vi "Test SwitchesMirrors.vi"() -> ()   [LabVIEW 2014]
uses:
  support/Instrument Status.ctl
  Spectrometer/Laser.ctl
  Spectrometer/Spectrometer Config.ctl
  Spectrometer/Laser Settings.ctl
  Spectrometer/Filter.ctl
  Spectrometer/Grating Detector Settings.ctl
  Spectrometer/Grating.ctl
  Spectrometer/Detector.ctl
  Spectrometer/Acquisition Settings.ctl
  SwitchesMirrors Config.ctl
  SwitchesMirrors Status.ctl
  SwitchesMirrors Refnum.ctl
  Camera/Camera Config.ctl
  Camera/Camera Settings.ctl
  Stress Control/StressControl Config.ctl
  Parameter Analyzer/Parameter Analyzer Config.ctl
  Parameter Analyzer/Parameter Analyzer Integration Parameters.ctl
  Parameter Analyzer/Parameter Analyzer SMU Sweeping.ctl
  Parameter Analyzer/Parameter Analyzer Sweep Spacing.ctl
  Parameter Analyzer/Parameter Analyzer SMU Range.ctl
  Parameter Analyzer/Parameter Analyzer SMU Sampling.ctl
  Parameter Analyzer/Parameter Analyzer Sampling Parameters.ctl
  Parameter Analyzer/Parameter Analyzer Stop Sampling Conditions.ctl
  Switching Matrix/Switching Matrix Config.ctl
  XYZ Stage/XYZ Config.ctl
  XYZ Stage/XYZ Connection Settings.ctl
  XYZ Stage/XYZ Stage Control.ctl
  XYZ Stage/XYZ Coordinate Control.ctl
  Autofocus/AutoFocus Config.ctl
  Autofocus/ZScan.ctl
  <vilib>/Analysis/Matrix/Datatypes/RealMatrix.ctl
  Measurements/Strain Measurement/Strain Measurement Config.ctl
  Measurements/Plot Data/PlotData Config.ctl
  Measurements/Plot Data/Measurement.ctl
  Measurements/Plot Data/WhichInstrument.ctl
  Parameter Analyzer/Electrical Data.ctl
  Spectrometer/Spectral Data.ctl
  Measurements/Instrument Sequence/Instrument Steps.ctl
  Measurements/Instrument Sequence/Action.ctl
  Measurements/Instrument Sequence/Instrument List.ctl
  support/User Event - Stop/User Event - Stop.lvlib
  support/Message Queue/Message Queue.lvlib
  <vilib>/Analysis/Matrix/NI_Matrix.lvlib
panel:
  out "Instrument Status":T1
  out "Status Log":string
  in  "Video":bool
  in  "Laser":bool
  in  "Switches & Mirrors VISA Session":refnum<visa-resource-name>="COM1"
  in  "Use LaserVideo Relays":bool=TRUE
  out "Last Operation":string
  in  "Exit":bool
  # "LICENSED MATERIALS – PROPERTY OF IBM\nCopyright IBM Corp. 2016,\nALL RIGHTS RESERVED"
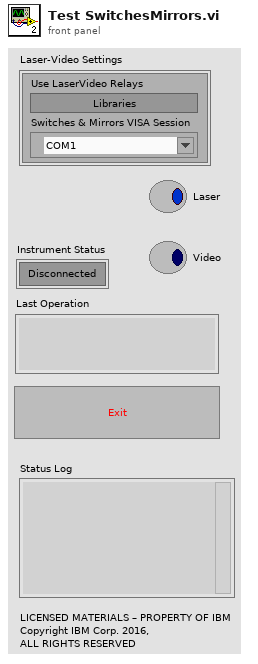
[diagram p1: front panel]
types:
  T1 = typedef "Instrument Status.ctl" = bool
  T2 = typedef "Message Queue.lvlib/All Message Queues.ctl" = cluster{"Message Handler Loop":refnum<queue>, "Parameter Analyzer":refnum<queue>, "Switching Matrix":refnum<queue>, "Stress Control":refnum<queue>, "Optical Spectrometer":refnum<queue>, "Switches & Mirrors":refnum<queue>, "Camera":refnum<queue>, "XYZ Stage":refnum<queue>, "AutoFocus":refnum<queue>, "Optoelectronic":refnum<queue>, "Save Data":refnum<queue>, "Plot Data":refnum<queue>, "Instrument Sequence":refnum<queue>, "Strain Measurement":refnum<queue>}
  T3 = typedef "Notifiers.ctl" = cluster{"Message Handler Loop":T4, "Parameter Analyzer":T5, "Switching Matrix":T6, "Stress Control":T7, "Optical Spectrometer":T8, "Switches & Mirrors":T9, "Camera":T10, "XYZ Stage":T11, "AutoFocus":T12, "Optoelectronic":T13, "Save Data":T14, "Plot Data":T14, "Instrument Sequence":T15, "Strain Measurement":cluster{"Status":refnum<notifier>, "Exit":refnum<notifier>, "Ready":refnum<notifier>}}
  T4 = typedef "Message Handler Loop Notifiers.ctl" = cluster{"Status":refnum<notifier>, "Instrument Data":refnum<notifier>, "Exit":refnum<notifier>, "Ready":refnum<notifier>}
  T5 = typedef "Parameter Analyzer Notifiers.ctl" = cluster{"Status":refnum<notifier>, "Instrument Data":refnum<notifier>, "Measurement":refnum<notifier>, "Exit":refnum<notifier>, "Ready":refnum<notifier>}
  T6 = typedef "Switching Matrix Notifiers.ctl" = cluster{"Status":refnum<notifier>, "Instrument Data":refnum<notifier>, "Measurement":refnum<notifier>, "Exit":refnum<notifier>, "Ready":refnum<notifier>}
  T7 = typedef "StressControl Notifiers.ctl" = cluster{"Status":refnum<notifier>, "Instrument Data":refnum<notifier>, "Measurement":refnum<notifier>, "Exit":refnum<notifier>, "Ready":refnum<notifier>}
  T8 = typedef "Spectrometer Notifiers.ctl" = cluster{"Status":refnum<notifier>, "Instrument Data":refnum<notifier>, "Measurement":refnum<notifier>, "Exit":refnum<notifier>, "Ready":refnum<notifier>}
  T9 = typedef "SwitchesMirrors Notifiers.ctl" = cluster{"Status":refnum<notifier>, "Instrument Data":refnum<notifier>, "Exit":refnum<notifier>, "Ready":refnum<notifier>}
  T10 = typedef "Camera Notifiers.ctl" = cluster{"Status":refnum<notifier>, "Instrument Data":refnum<notifier>, "Measurement":refnum<notifier>, "Exit":refnum<notifier>, "Ready":refnum<notifier>}
  T11 = typedef "XYZ Notifications.ctl" = cluster{"Status":refnum<notifier>, "Instrument Data":refnum<notifier>, "Measurement":refnum<notifier>, "Exit":refnum<notifier>, "Ready":refnum<notifier>}
  T12 = typedef "Autofocus Notifiers.ctl" = cluster{"Status":refnum<notifier>, "Instrument Data":refnum<notifier>, "Measurement":refnum<notifier>, "Exit":refnum<notifier>, "Ready":refnum<notifier>}
  T13 = typedef "Optoelectronic Notifiers.ctl" = cluster{"Status":refnum<notifier>, "Instrument Data":refnum<notifier>, "Measurement":refnum<notifier>, "Exit":refnum<notifier>, "Ready":refnum<notifier>}
  T14 = typedef "SaveData Notifiers.ctl" = cluster{"Status":refnum<notifier>, "Exit":refnum<notifier>, "Ready":refnum<notifier>}
  T15 = typedef "Instrument Sequence Notifiers.ctl" = cluster{"Status":refnum<notifier>, "Instrument Data":refnum<notifier>, "Measurement":refnum<notifier>, "Exit":refnum<notifier>, "Ready":refnum<notifier>}
  T16 = typedef "Configuration.ctl" = cluster{"Parameter Analizer":T17, "Switching Matrix":T25, "Stress Control":T26, "Optical Spectrometer":T27, "Switches & Mirrors":T35, "Camera":T37, "XYZ Stage":T39, "AutoFocus":T43, "Sava Data":T46, "PlotData":T51, "Instrument Sequence":T57, "Strain Measurement":T58}
  T17 = typedef "Parameter Analyzer Config.ctl" = cluster{"Parameter Analyzer VISA Session":refnum<visa-resource-name>, "Sweeping Time Parameters":T18, "Acquisition Mode":enum32{"Sweeping Mode", "Sampling Mode"}, "Status Polling Time (ms)":u32, "Comment":string, "SMU 1 - Sweeping":T19, "SMU 2 - Sweeping":T19, "SMU 3 - Sweeping":T19, "SMU 4 - Sweeping":T19, "Sweep Spacing":T20, "Range":T21, "SMU1 - Sampling":T22, "SMU2 - Sampling":T22, "SMU3 - Sampling":T22, "SMU4 - Sampling":T22, "Sampling Time Parameters":T23, "Stop Condition":T24}
  T18 = typedef "Parameter Analyzer Integration Parameters.ctl" = cluster{"Integration Time":u32, "Short Integration Time (s)":dbl, "Long Integration Time (s)":dbl, "Wait Time Parameter":dbl}
  T19 = typedef "Parameter Analyzer SMU Sweeping.ctl" = cluster{"Start / Offset":dbl, "Stop / Ratio":dbl, "Step \n(linear only)":dbl, "Compliance":dbl, "Power \nCompliance":dbl, "Mode":u32, "Function":i32, "Sweep Mode":bool}
  T20 = typedef "Parameter Analyzer Sweep Spacing.ctl" = u16
  T21 = typedef "Parameter Analyzer SMU Range.ctl" = u16
  T22 = typedef "Parameter Analyzer SMU Sampling.ctl" = cluster{"Source":dbl, "Compliance":dbl, "Mode":u32, "Function":bool}
  T23 = typedef "Parameter Analyzer Sampling Parameters.ctl" = cluster{"Initial Interval (s)":dbl, "Number of Samples":i32, "Total Sampling Time (s)":dbl, "Hold Time (s)":dbl, "Sampling Mode":i32, "Sampling Time":i32}
  T24 = typedef "Parameter Analyzer Stop Sampling Conditions.ctl" = cluster{"Enable Delay (s)":dbl, "Name":string, "Threshold":dbl, "num. of events":i32, "Event":i32, "Stop Condition Enable":bool}
  T25 = typedef "Switching Matrix Config.ctl" = cluster{"Switching Matrix VISA Session":refnum<visa-resource-name>, "Connections":cluster{"Connections":bool[], "Connection Type":enum16{"Disconnected", "Make - Break", "Break - Make"}}[]}
  T26 = typedef "StressControl Config.ctl" = cluster{"Stress Control VISA Session":refnum<visa-resource-name>, "Axis":i32, "Motion":u16, "Destination (°)":dbl, "Speed (°/s)":dbl, "Position (°)":dbl}
  T27 = typedef "Spectrometer Config.ctl" = cluster{"Laser Settings":T28, "Spectrometer Settings":T31, "Acquisition Settings":T34, "Path":path}
  T28 = typedef "Laser Settings.ctl" = cluster{"Laser Wavelength":T29, "Neutral Density Filter":T30}
  T29 = typedef "Laser.ctl" = enum16{"633 nm", "784 nm", "532 nm", "365 nm"}
  T30 = typedef "Filter.ctl" = enum16{"100%", "50%", "25%", "10%", "1%", "0.1%", "0.01%"}
  T31 = typedef "Grating Detector Settings.ctl" = cluster{"Confocal Hole Size (µm)":dbl, "Grating":T32, "Detector":T33}
  T32 = typedef "Grating.ctl" = u16
  T33 = typedef "Detector.ctl" = enum16{"InGaAs Array", "Silicon CCD"}
  T34 = typedef "Acquisition Settings.ctl" = cluster{"Acquisition Mode":enum16{"Single Window", "Multi-Window"}, "Spectal Position (nm)":dbl, "From (nm)":dbl, "To (nm)":dbl, "Integration Time (s)":dbl, "Number of Accumulations":i32, "AutoScanning":bool, "Spike Removal":bool}
  T35 = typedef "SwitchesMirrors Config.ctl" = cluster{"Relay VISA Session":refnum<visa-resource-name>, "Switches":T36, "Delays (ms)":cluster{"Laser":u32, "Video":u32}}
  T36 = typedef "SwitchesMirrors Status.ctl" = cluster{"Laser":bool, "Video":bool}
  T37 = typedef "Camera Config.ctl" = cluster{"Settings":T38}
  T38 = typedef "Camera Settings.ctl" = cluster{"Pixel clock":i32, "Frame rate":dbl, "Exposure time":dbl, "Master Gain":i32, "Red Gain":i32, "Green Gain":i32, "Blue Gain":i32, "Auto Gain":bool, "White-balance":bool, "Color Correction":bool}
  T39 = typedef "XYZ Config.ctl" = cluster{"Connection Settings":T40, "Manual Control":T41, "Coordinate Control":T42}
  T40 = typedef "XYZ Connection Settings.ctl" = cluster{"Tango VISA":refnum<visa-resource-name>, "Baudrate":i32, "Show Protocol?":bool}
  T41 = typedef "XYZ Stage Control.ctl" = cluster{"North":bool, "South":bool, "West":bool, "East":bool, "Up":bool, "Down":bool, "Stop":bool, "XY Step":dbl, "Z step":dbl}
  T42 = typedef "XYZ Coordinate Control.ctl" = cluster{"Motion Mode":enum16{"Absolute", "Relative"}, "Destination [mm]":dbl[]}
  T43 = typedef "AutoFocus Config.ctl" = cluster{"Matching Criteria":cluster{"Minimum Score":sgl, "Color Score Weight":sgl, "Minimum Contrast":i32, "Match Mode":u32, "Match Feature Mode":u32, "Subpixel Accuracy":bool, "Color Sensitivity":u32, "Search Strategy":u32}, "Z Scan Parameters":T44, "Displacement":dbl, "Transformation Matrix":T45}
  T44 = typedef "ZScan.ctl" = cluster{"Z Range":ext, "Resolution":dbl, "Initial Direction":enum16{"Up", "Down"}, "Focus Threshold":dbl, "Ascent Constant":dbl}
  T45 = typedef "NI_Matrix.lvlib/RealMatrix.ctl" = dbl[][]
  T46 = typedef "SaveData Config.ctl" = cluster{"Workspace Info":T47, "Instrument Configuration":T48, "Stress Motor Position":dbl, "Electrical Measurement":cluster{"Sequence":dbl[], "V1":dbl[], "V2":dbl[], "V3":dbl[], "V4":dbl[], "I1":dbl[], "I2":dbl[], "I3":dbl[], "I4":dbl[]}, "Optical Spectrum":T50}
  T47 = typedef "SaveData Workspace Info.ctl" = cluster{"Device Name":string, "Device Info":string, "Path":path}
  T48 = typedef "SaveData Instrument Configuration.ctl" = cluster{"Instrument":T49, "Configuration":string}
  T49 = typedef "Instrument List.ctl" = enum32{"Unknown Instrument", "Switching Matrix", "Parameter Analyzer", "Optical Spectrometer", "Optoelectronic", "Autofocus"}
  T50 = typedef "Spectral Data.ctl" = cluster{"Intensity":dbl[], "Wavelength":dbl[], "Energy":dbl[], "Raman Shift":dbl[], "Detector Temperature":dbl}
  T51 = typedef "PlotData Config.ctl" = cluster{"Sliders":cluster{"Strain Sequence":i32, "Instrument Sequence":i32}, "Measurement":T52, "Instrument Steps":T55, "Strain Points":dbl[]}
  T52 = typedef "Measurement.ctl" = cluster{"Which Instrument?":T53, "Electrical Measurement":T54, "Measurement Mode":enum16{"Sweeping Mode", "Sampling Mode"}, "Optical Spectrum":T50}
  T53 = typedef "WhichInstrument.ctl" = enum16{"No Plot", "Spectrometer", "Parameter Analyzer", "Optoelectronic"}
  T54 = typedef "Electrical Data.ctl" = cluster{"Sequence":dbl[], "V1":dbl[], "V2":dbl[], "V3":dbl[], "V4":dbl[], "I1":dbl[], "I2":dbl[], "I3":dbl[], "I4":dbl[]}
  T55 = typedef "Instrument Steps.ctl" = cluster{"Action":T56, "Configuration":variant, "Instrument":T49, "Status":enum8{"False", "True", "Mixed"}}[]
  T56 = typedef "Action.ctl" = enum32{"Configure", "Measure"}
  T57 = typedef "Instrument Sequence Config.ctl" = cluster{"Caller VI":enum16{"User", "Stress Measurement VI"}}
  T58 = typedef "Strain Measurement Config.ctl" = cluster{"Stress Sequence ":cluster{"Max Motor Position":ext, "# Intermediate Points":u32, "Initial Direction":enum16{"Tension", "Compression"}}, "Track?":bool}
  T59 = typedef "SwitchesMirrors Refnum.ctl" = cluster{"Instrument Status":refnum<vi>, "Laser":refnum<vi>, "Video":refnum<vi>, "Relay VISA":refnum<vi>}
  T60 = cluster{"SMU 1 - Sweeping":cluster{"Start / Offset":dbl, "Stop / Ratio":dbl, "Step (linear only)":dbl, "Compliance":dbl, "Power Compliance":dbl, "Mode":u32, "Function":i32, "Sweep Mode":bool}, "SMU 2 - Sweeping":cluster{"Start / Offset":dbl, "Stop / Ratio":dbl, "Step (linear only)":dbl, "Compliance":dbl, "Power Compliance":dbl, "Mode":u32, "Function":i32, "Sweep Mode":bool}, "SMU 3 - Sweeping":cluster{"Start / Offset":dbl, "Stop / Ratio":dbl, "Step (linear only)":dbl, "Compliance":dbl, "Power Compliance":dbl, "Mode":u32, "Function":i32, "Sweep Mode":bool}, "SMU 4 - Sweeping":cluster{"Start / Offset":dbl, "Stop / Ratio":dbl, "Step (linear only)":dbl, "Compliance":dbl, "Power Compliance":dbl, "Mode":u32, "Function":i32, "Sweep Mode":bool}, "Sweep Spacing":u16, "Range":u16}
  T61 = cluster{"SMU1 - Sampling":cluster{"Source":dbl, "Compliance":dbl, "Mode":u32, "Function":bool}, "SMU2 - Sampling":cluster{"Source":dbl, "Compliance":dbl, "Mode":u32, "Function":bool}, "SMU3 - Sampling":cluster{"Source":dbl, "Compliance":dbl, "Mode":u32, "Function":bool}, "SMU4 - Sampling":cluster{"Source":dbl, "Compliance":dbl, "Mode":u32, "Function":bool}, "Sampling Parameters":cluster{"Initial Interval (s)":dbl, "Number of Samples":i32, "Total Sampling Time (s)":dbl, "Hold Time (s)":dbl, "Sampling Mode":i32, "Sampling Time":i32}, "Stop Condition":cluster{"Enable Delay (s)":dbl, "Name":string, "Threshold":dbl, "num. of events":i32, "Event":i32, "Stop Condition Enable":bool}}
  T62 = cluster{"PlotData - Instrument Sequence":i32, "PlotData - Strain Sequence":i32}
  T63 = cluster{"Start / Offset":dbl, "Stop / Ratio":dbl, "Step (linear only)":dbl, "Compliance":dbl, "Power Compliance":dbl, "Mode":u32, "Function":i32, "Sweep Mode":bool}
  T64 = cluster{"Source":dbl, "Compliance":dbl, "Mode":u32, "Function":bool}
  T65 = cluster{"Initial Interval (s)":dbl, "Number of Samples":i32, "Total Sampling Time (s)":dbl, "Hold Time (s)":dbl, "Sampling Mode":i32, "Sampling Time":i32}
  T66 = cluster{"Enable Delay (s)":dbl, "Name":string, "Threshold":dbl, "num. of events":i32, "Event":i32, "Stop Condition Enable":bool}
  T67 = cluster{"Connections":bool[], "Connection Type":enum16{"Disconnected", "Make - Break", "Break - Make"}}[]
  T68 = cluster{"Minimum Score":sgl, "Color Score Weight":sgl, "Minimum Contrast":i32, "Match Mode":u32, "Match Feature Mode":u32, "Subpixel Accuracy":bool, "Color Sensitivity":u32, "Search Strategy":u32}
  T69 = cluster{"Max Motor Position":ext, "# Intermediate Points":u32, "Initial Direction":enum16{"Tension", "Compression"}}
  T70 = enum32{"invalid app kind", "Development System", "Run Time System", "Student Edition", "Embedded LabVIEW", "Evaluation", "Custom"}
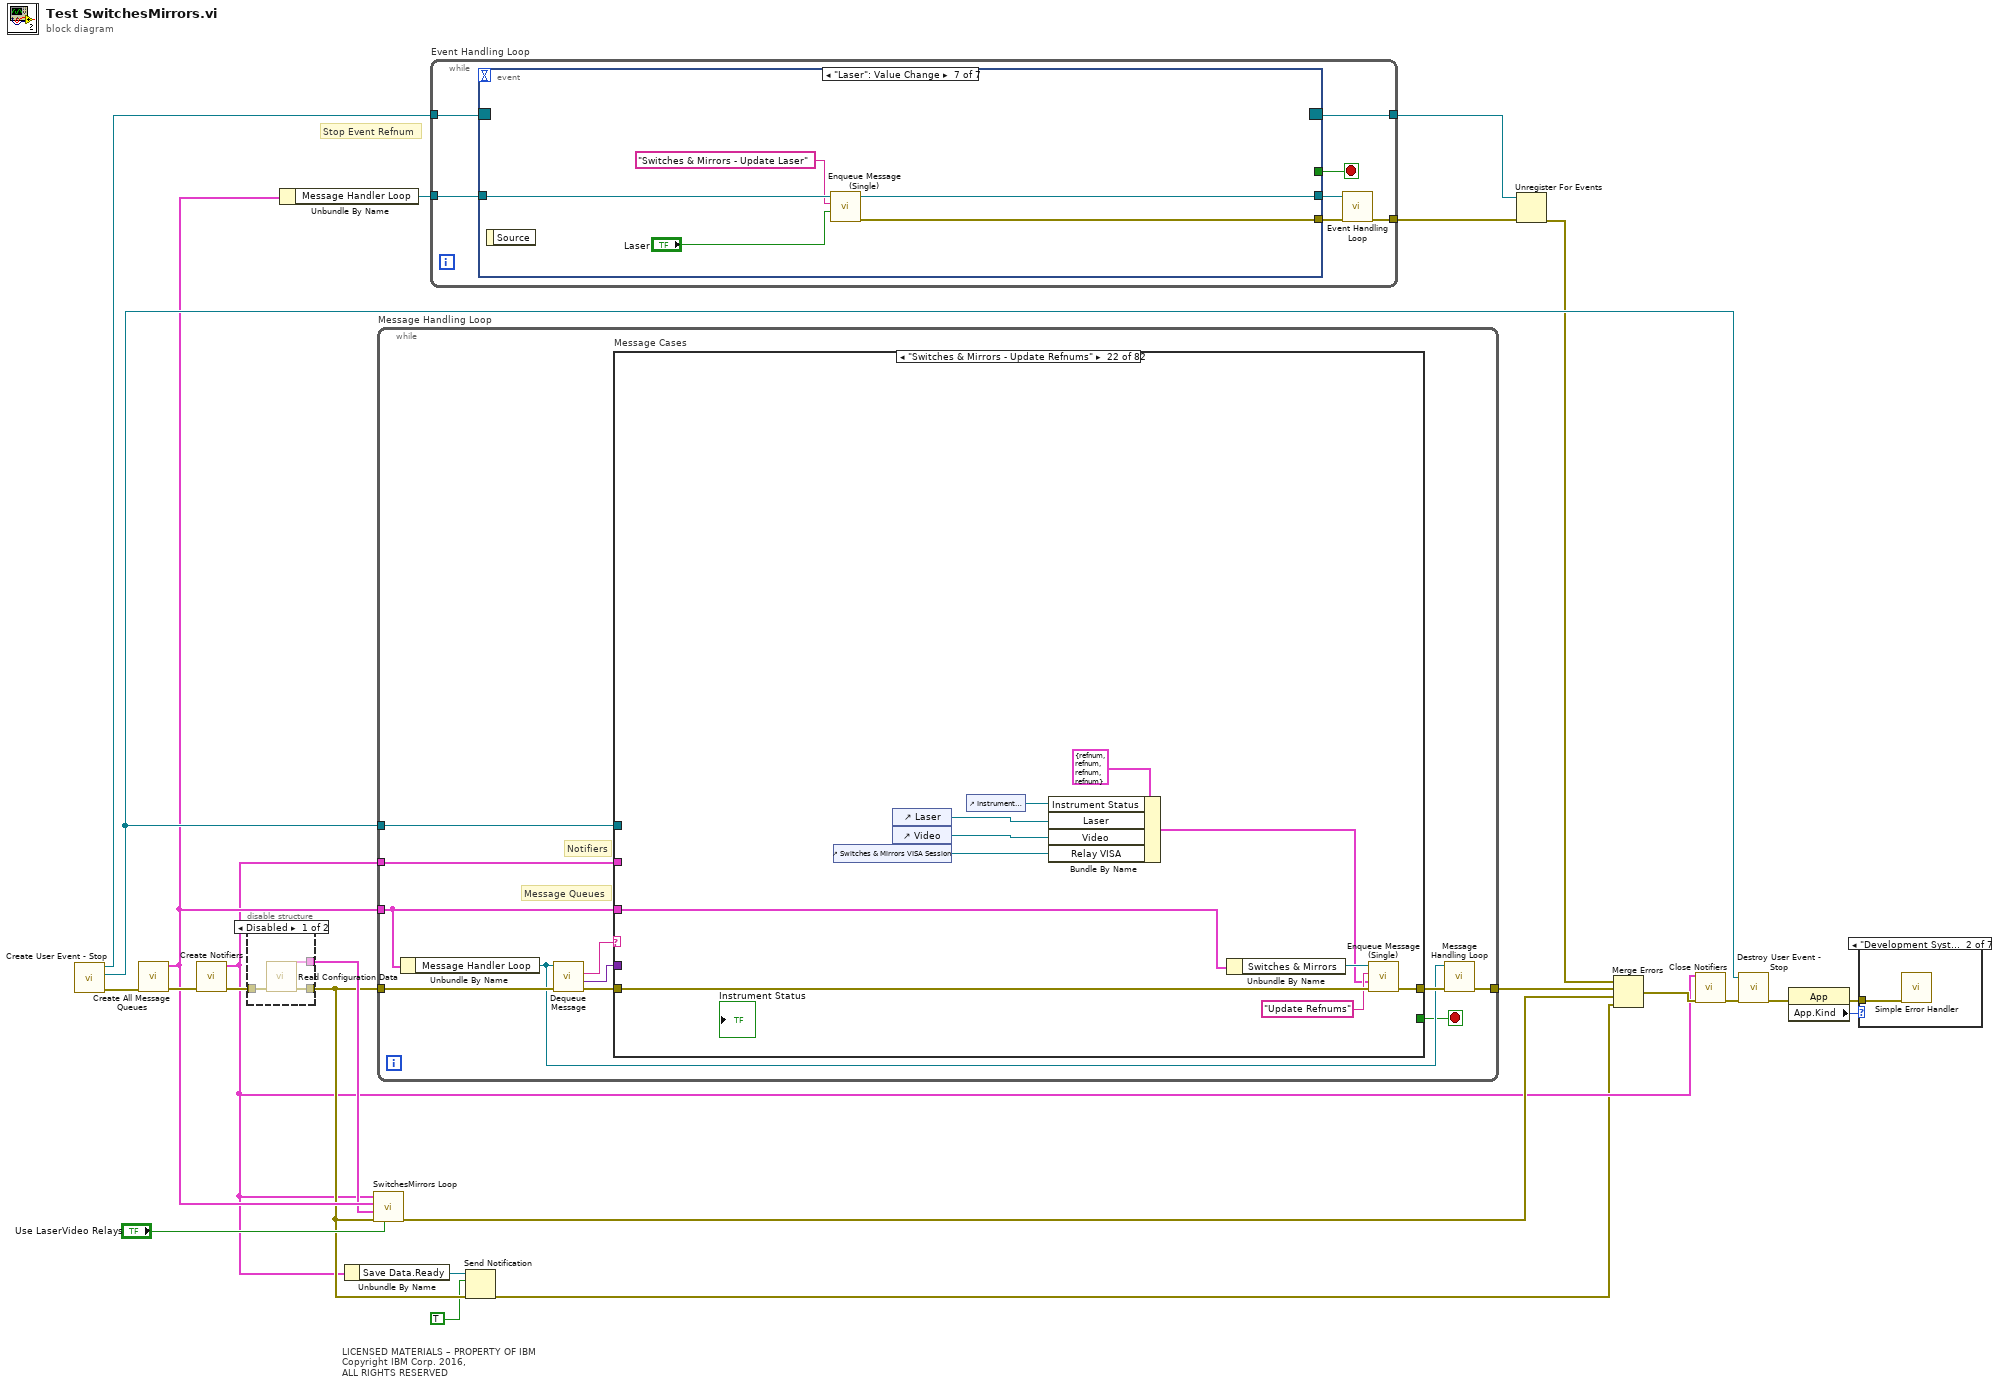
[diagram p0: block diagram]
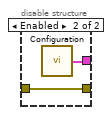
[diagram p2: hidden frame]
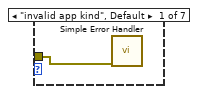
[diagram p3: hidden frame]
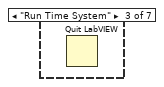
[diagram p4: hidden frame]
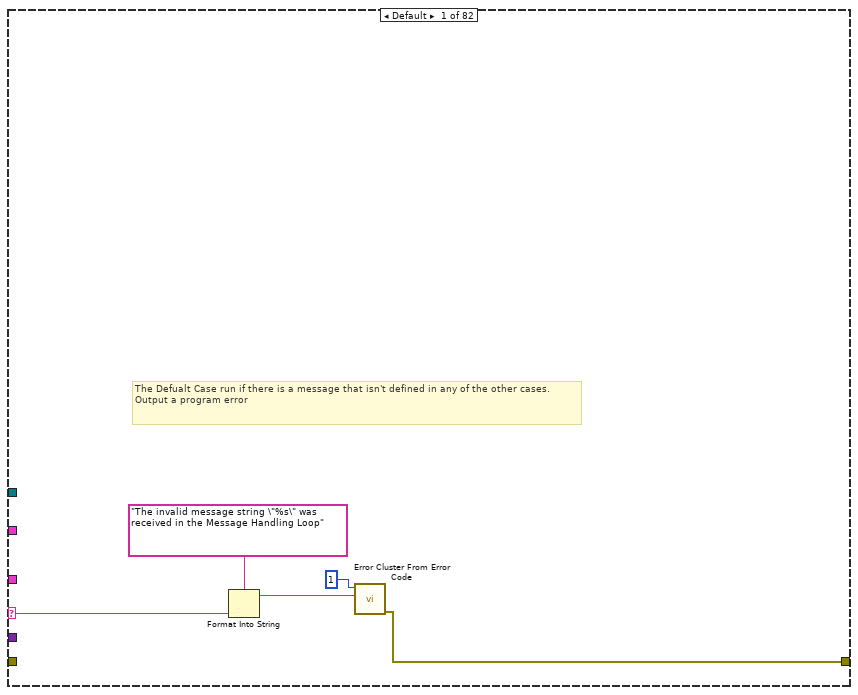
[diagram p9: hidden frame]
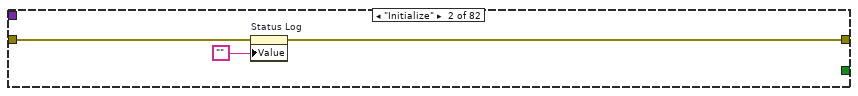
[diagram p10: hidden frame]
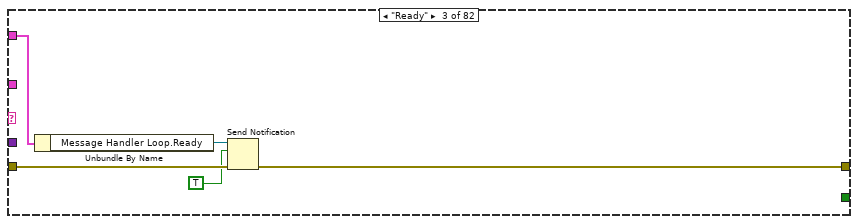
[diagram p11: hidden frame]
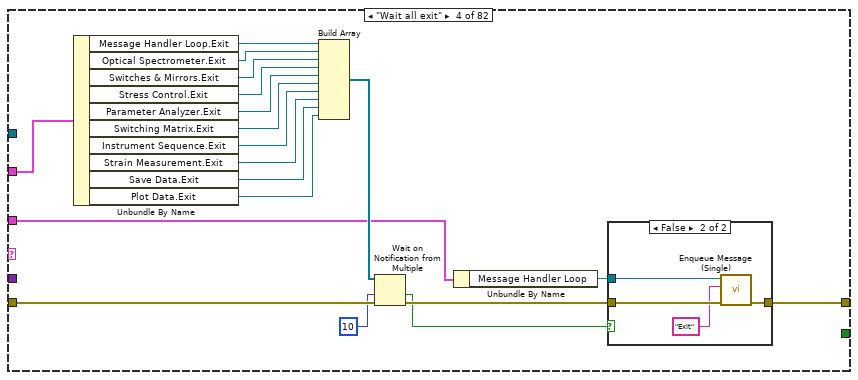
[diagram p12: hidden frame]
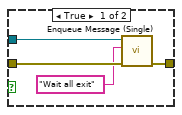
[diagram p13: hidden frame]
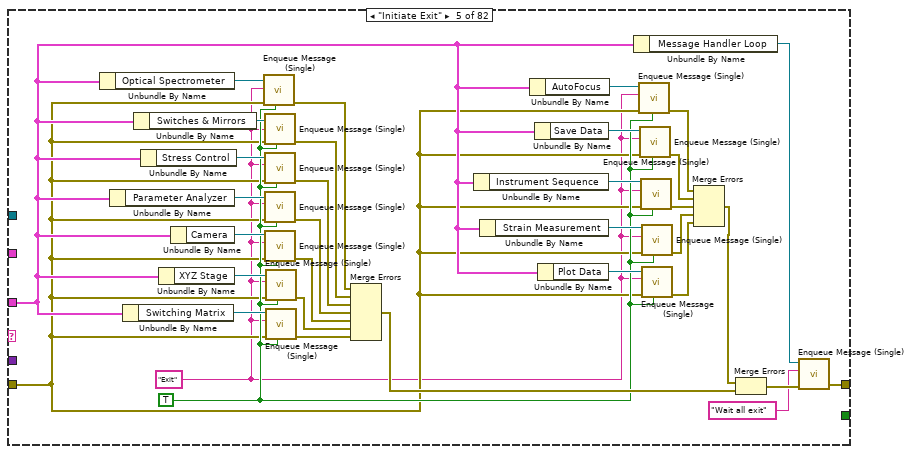
[diagram p14: hidden frame]
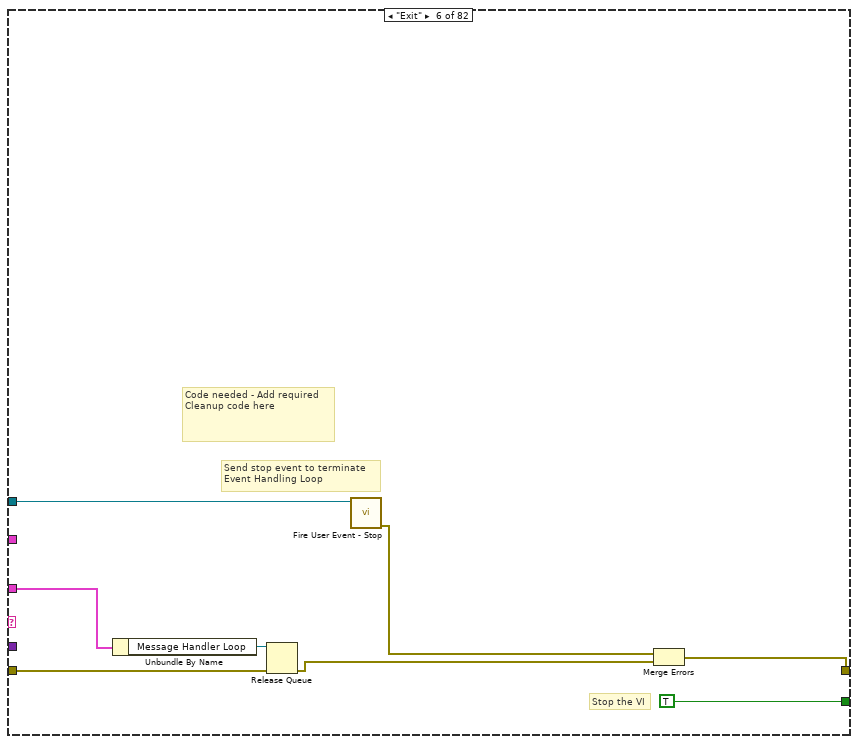
[diagram p15: hidden frame]
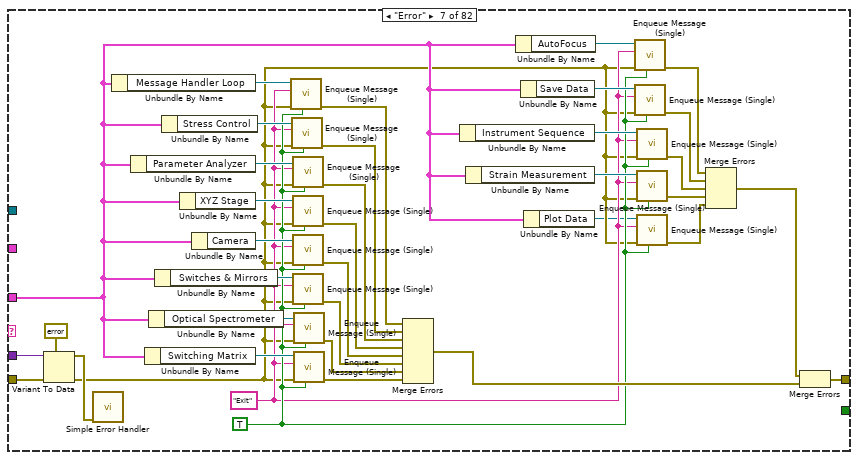
[diagram p16: hidden frame]
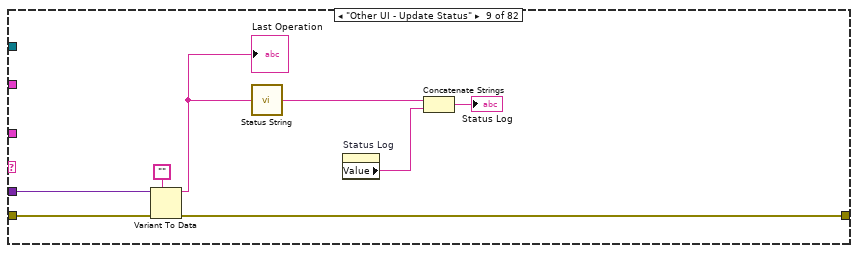
[diagram p18: hidden frame]
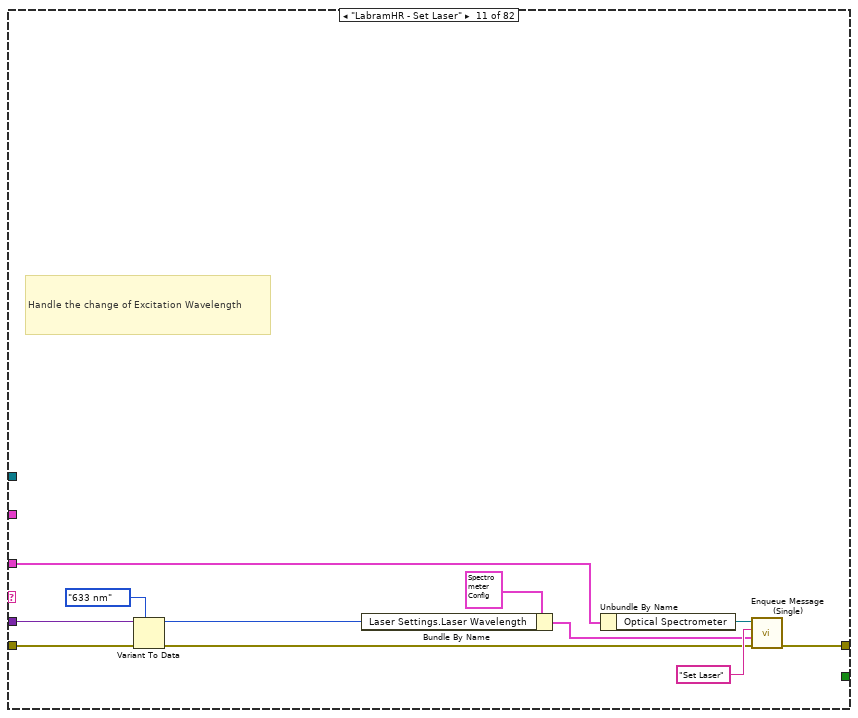
[diagram p20: hidden frame]
diagram:
  # "LICENSED MATERIALS – PROPERTY OF IBM\nCopyright IBM Corp. 2016,\nALL RIGHTS RESERVED"
  # "Stop Event Refnum"
  n1 = call "Create User Event - Stop.vi"() -> ("error out"=w14:errorcluster, "User Event - Stop"=w17:refnum<user-event>, "Stop Event Registration Refnum"=w24:refnum<event-registration>)  [unwired: 1 in, 8 out]
  n2 = call "Create All Message Queues.vi"("error in (no error)"=w14) -> ("error out"=w13:errorcluster, "Message Queues out"=w10:T2)  [unwired: 9 out]
  n3 = call "Create Notifiers.vi"("error in"=w13) -> ("error out"=w12:errorcluster, "Notifiers"=w4:T3)  [unwired: 9 out]
  n4 = disable-structure shown="Disabled" {
    disable-tunnel: w12 -> [w27 w29]
    disable-tunnel: [w26 w29] -> w5
    disable-tunnel: [w25 w28] -> w6
    frame Disabled {
      n5 = call "Read Configuration Data.vi"("error in"=w27) -> ("error out"=w26:errorcluster, "System Configuration"=w25:T16)  [unwired: 9 out]
    }
    frame Enabled {
      n6 = call "Configuration.vi"() -> ("IBM OptoElectroMechanics Configuration"=w28:T16)
    }
  }
  n7 = Unbundle By Name(w10) -> ("Message Handler Loop"=w22:refnum<queue>)
  n8 = Unbundle By Name(w4) -> ("Save Data.Ready"=w3:refnum<notifier>)
  n9 = call "SwitchesMirrors Loop.vi"("Used functions"="Use LaserVideo Relays", "error in"=w5, "IBM OptoElectroMechanics Configuration"=w6, "Message Queues out"=w10, "Notifiers"=w4) -> ("error out"=w7:errorcluster)  [unwired: 6 out]
  n10 = while "Message Handling Loop" {
    tunnel: w5 -> [w40]
    tunnel: [w37] -> w8
    tunnel: w10 -> [w31]
    tunnel: w17 -> [w33]
    tunnel: w4 -> [w30]
    stop <- w32 stop-if-true
    # "Notifiers"
    # "Message Queues"
    n11 = Unbundle By Name(w31) -> ("Message Handler Loop"=w36:refnum<queue>)
    n12 = call "Dequeue Message.vi"("error in (no error)"=w40, "Message Queue"=w36) -> ("error out"=w39:errorcluster, "Message Data"=w34:variant, "Message"=w35:string)  [unwired: 7 out]
    n13 = case "Message Cases" shown="\"Switches & Mirrors - Update Refnums\"" w35 {
      selector: w35 -> [w45 _ _ _ _ _ _ _ _ _ _ _ _ _ _ _ _ _ _ _ _ _ _ _ _ _ _ _ _ _ _ _ _ _ _ _ _ _ _ _ _ _ _ _ _ _ _ _ _ _ _ _ _ _ _ _ _ _ _ _ _ _ _ _ _ _ _ _ _ _ _ _ _ _ _ _ _ _ _ _ _ _]
      tunnel: w39 -> [_ w47 w52 w71 w84 w121 w148 w160 w168 w169 w176 w191 w202 w213 w224 w235 w246 w250 w255 w257 w265 w270 w284 w297 w308 w310 w320 w322 w327 w332 w343 w354 w355 w360 w364 w375 w386 w403 w420 w421 w426 w434 w445 w449 w454 w459 w470 w481 w482 w493 w504 w515 w516 w521 w526 w531 w536 w541 w546 w551 w556 w559 w564 w569 w574 w579 w582 w587 w592 w597 w608 w613 w618 w623 w626 w631 w636 w641 w646 w649 w662 w663]
      tunnel: [w41 w46 w53 w60 w100 w122 w157 w160 w165 w169 w174 w187 w198 w210 w221 w231 w244 w247 w252 w257 w261 w276 w287 w296 w307 w310 w319 w326 w331 w332 w342 w353 w359 w360 w363 w369 w381 w392 w412 w423 w426 w437 w448 w453 w458 w459 w465 w477 w482 w488 w499 w510 w519 w524 w529 w534 w539 w544 w549 w554 w556 w558 w563 w568 w573 w578 w584 w589 w594 w597 w605 w612 w617 w622 w625 w630 w635 w640 w645 w649 w657 w663] -> w38
      tunnel: w34 -> [_ _ _ _ _ _ w159 _ w167 _ w180 w190 w201 w212 w223 w234 w245 _ _ _ w260 _ w280 w298 w309 _ w321 _ _ _ w337 w348 _ _ w362 w374 w385 w402 w419 _ _ w431 w442 _ _ _ w469 w480 _ w492 w503 w514 _ _ _ _ _ _ _ _ _ _ _ _ _ _ _ _ _ _ w607 _ _ _ _ _ _ _ _ _ w661 _]
      tunnel: w33 -> [_ _ _ _ _ w119 _ _ _ _ _ _ _ _ _ _ _ _ _ _ _ _ _ _ _ _ _ _ _ _ _ _ _ _ _ _ _ _ _ _ _ _ _ _ _ _ _ _ _ _ _ _ _ _ _ _ _ _ _ _ _ _ _ _ _ _ _ _ _ _ _ _ _ _ _ _ _ _ _ _ _ _]
      tunnel: [_ _ _ _ _ TRUE _ _ _ _ _ _ _ _ _ _ _ _ _ _ _ _ _ _ _ _ _ _ _ _ _ _ _ _ _ _ _ _ _ _ _ _ _ _ _ _ _ _ _ _ _ _ _ _ _ _ _ _ _ _ _ _ _ _ _ _ _ _ _ _ _ _ _ _ _ _ _ _ _ _ _ _] -> w32
      tunnel: w31 -> [_ _ _ w59 w87 w116 w129 _ _ _ w179 w186 w195 w208 w219 w228 w240 w248 w253 _ _ w274 w285 w293 w304 _ w317 w324 w329 _ w339 w350 w357 _ _ w371 w380 w391 w411 w422 _ w435 w446 w451 w456 _ w464 w476 _ w487 w498 w509 w518 w523 w528 w533 w538 w543 w548 w553 _ w561 w566 w571 w576 w581 w586 w591 w596 _ w602 w609 w614 w619 w628 w633 w638 w643 w648 _ w656 _]
      tunnel: w30 -> [_ _ w51 w72 _ _ _ _ _ _ _ _ _ _ _ _ _ _ _ _ _ _ _ _ _ _ _ _ _ _ _ _ _ _ _ _ _ _ _ _ _ _ _ _ _ _ _ _ _ _ _ _ _ _ _ _ _ _ _ _ _ _ _ _ _ _ _ _ _ _ _ _ _ _ _ _ _ _ _ _ _ _]
      frame Default {
        # "The Defualt Case run if there is a message that isn't defined in any of the other cases.\nOutput a program error"
        n14 = Format Into String(format string="The invalid message string \"%s\" was  received in the Message Handling Loop", w45) -> (resulting string=w43:string)  [unwired: 2 in, 1 out]
        n15 = call <vilib>:"Error Cluster From Error Code.vi"("error message (\"\")"=w43, "error code (0)"=1) -> ("error out"=w41:errorcluster)  [unwired: 2 in, 5 out]
      }
      frame "Initialize" {
        n16 = property on="Status Log" class="Str"(error in=w47, "Value"="") -> (error out=w46:errorcluster)  [unwired: 1 in, 1 out]
      }
      frame "Ready" {
        n17 = Unbundle By Name(w51) -> ("Message Handler Loop.Ready"=w50:refnum<notifier>)
        n18 = Send Notification(notification=TRUE, notifier=w50, error in (no error)=w52) -> (error out=w53:errorcluster)  [unwired: 1 out]
      }
      frame "Wait all exit" {
        n19 = Unbundle By Name(w72) -> ("Message Handler Loop.Exit"=w69:refnum<notifier>, "Optical Spectrometer.Exit"=w68:refnum<notifier>, "Switches & Mirrors.Exit"=w67:refnum<notifier>, "Stress Control.Exit"=w66:refnum<notifier>, "Parameter Analyzer.Exit"=w65:refnum<notifier>, "Switching Matrix.Exit"=w64:refnum<notifier>, "Instrument Sequence.Exit"=w57:refnum<notifier>, "Strain Measurement.Exit"=w56:refnum<notifier>, "Save Data.Exit"=w55:refnum<notifier>, "Plot Data.Exit"=w54:refnum<notifier>)
        n20 = Build Array(w69, w68, w67, w66, w65, w64, w57, w56, w55, w54) -> (w63:refnum<notifier>[])
        n21 = Wait on Notification from Multiple(0:w63, 2:10 ("timeout in ms (-1)"), 3:w71) -> (10:w58:bool, 11:w61:errorcluster)  [unwired: 3 out]
        n22 = Unbundle By Name(w59) -> ("Message Handler Loop"=w62:refnum<queue>)
        n23 = case shown="False" w58 {
          tunnel: w62 -> [w76 w80]
          tunnel: w61 -> [w75 w79]
          tunnel: [w74 w78] -> w60
          frame True {
            n24 = call "Enqueue Message (Single).vi"("error in (no error)"=w75, "Message"="Wait all exit", "Message Queue"=w76) -> ("error out"=w74:errorcluster)  [unwired: 1 in, 7 out]
          }
          frame False {
            n25 = call "Enqueue Message (Single).vi"("error in (no error)"=w79, "Message"="Exit", "Message Queue"=w80) -> ("error out"=w78:errorcluster)  [unwired: 1 in, 7 out]
          }
        }
      }
      frame "Initiate Exit" {
        w85 = TRUE ("Priority Message? (F)")
        w82 = "Exit" ("Message")
        n26 = Unbundle By Name(w87) -> ("Optical Spectrometer"=w104:refnum<queue>)
        n27 = Unbundle By Name(w87) -> ("Parameter Analyzer"=w101:refnum<queue>)
        n28 = Unbundle By Name(w87) -> ("Switching Matrix"=w96:refnum<queue>)
        n29 = Unbundle By Name(w87) -> ("Switches & Mirrors"=w103:refnum<queue>)
        n30 = Unbundle By Name(w87) -> ("Stress Control"=w102:refnum<queue>)
        n31 = Unbundle By Name(w87) -> ("XYZ Stage"=w114:refnum<queue>)
        n32 = Unbundle By Name(w87) -> ("Camera"=w105:refnum<queue>)
        n33 = call "Enqueue Message (Single).vi"("Priority Message? (F)"=w85, "error in (no error)"=w84, "Message"=w82, "Message Queue"=w104) -> ("error out"=w106:errorcluster)  [unwired: 1 in, 6 out]
        n34 = call "Enqueue Message (Single).vi"("Priority Message? (F)"=w85, "error in (no error)"=w84, "Message"=w82, "Message Queue"=w103) -> ("error out"=w107:errorcluster)  [unwired: 1 in, 6 out]
        n35 = call "Enqueue Message (Single).vi"("Priority Message? (F)"=w85, "error in (no error)"=w84, "Message"=w82, "Message Queue"=w102) -> ("error out"=w108:errorcluster)  [unwired: 1 in, 6 out]
        n36 = call "Enqueue Message (Single).vi"("Priority Message? (F)"=w85, "error in (no error)"=w84, "Message"=w82, "Message Queue"=w101) -> ("error out"=w109:errorcluster)  [unwired: 1 in, 6 out]
        n37 = call "Enqueue Message (Single).vi"("Priority Message? (F)"=w85, "error in (no error)"=w84, "Message"=w82, "Message Queue"=w105) -> ("error out"=w110:errorcluster)  [unwired: 1 in, 6 out]
        n38 = call "Enqueue Message (Single).vi"("Priority Message? (F)"=w85, "error in (no error)"=w84, "Message"=w82, "Message Queue"=w114) -> ("error out"=w111:errorcluster)  [unwired: 1 in, 6 out]
        n39 = call "Enqueue Message (Single).vi"("Priority Message? (F)"=w85, "error in (no error)"=w84, "Message"=w82, "Message Queue"=w96) -> ("error out"=w112:errorcluster)  [unwired: 1 in, 6 out]
        n40 = Merge Errors(w106, w107, w108, w109, w110, w111, w112) -> (w113:errorcluster)
        n41 = Unbundle By Name(w87) -> ("Instrument Sequence"=w93:refnum<queue>)
        n42 = Unbundle By Name(w87) -> ("Strain Measurement"=w89:refnum<queue>)
        n43 = Unbundle By Name(w87) -> ("AutoFocus"=w95:refnum<queue>)
        n44 = Unbundle By Name(w87) -> ("Save Data"=w94:refnum<queue>)
        n45 = Unbundle By Name(w87) -> ("Plot Data"=w86:refnum<queue>)
        n46 = Unbundle By Name(w87) -> ("Message Handler Loop"=w98:refnum<queue>)
        n47 = call "Enqueue Message (Single).vi"("Priority Message? (F)"=w85, "error in (no error)"=w84, "Message"=w82, "Message Queue"=w95) -> ("error out"=w92:errorcluster)  [unwired: 1 in, 6 out]
        n48 = call "Enqueue Message (Single).vi"("Priority Message? (F)"=w85, "error in (no error)"=w84, "Message"=w82, "Message Queue"=w94) -> ("error out"=w91:errorcluster)  [unwired: 1 in, 6 out]
        n49 = call "Enqueue Message (Single).vi"("Priority Message? (F)"=w85, "error in (no error)"=w84, "Message"=w82, "Message Queue"=w93) -> ("error out"=w90:errorcluster)  [unwired: 1 in, 6 out]
        n50 = call "Enqueue Message (Single).vi"("Priority Message? (F)"=w85, "error in (no error)"=w84, "Message"=w82, "Message Queue"=w89) -> ("error out"=w88:errorcluster)  [unwired: 1 in, 6 out]
        n51 = call "Enqueue Message (Single).vi"("Priority Message? (F)"=w85, "error in (no error)"=w84, "Message"=w82, "Message Queue"=w86) -> ("error out"=w83:errorcluster)  [unwired: 1 in, 6 out]
        n52 = Merge Errors(w92, w91, w90, w88, w83) -> (w81:errorcluster)
        n53 = Merge Errors(w81, w113) -> (w99:errorcluster)
        n54 = call "Enqueue Message (Single).vi"("error in (no error)"=w99, "Message"="Wait all exit", "Message Queue"=w98) -> ("error out"=w100:errorcluster)  [unwired: 1 in, 7 out]
      }
      frame "Exit" {
        # "Send stop event to terminate \nEvent Handling Loop"
        # "Stop the VI"
        # "Code needed - Add required Cleanup code here"
        n55 = Unbundle By Name(w116) -> ("Message Handler Loop"=w115:refnum<queue>)
        n56 = Release Queue(queue=w115, error in (no error)=w121) -> (error out=w120:errorcluster)  [unwired: 3 out]
        n57 = call "Fire User Event - Stop.vi"("User Event - Stop"=w119) -> ("error out"=w118:errorcluster)  [unwired: 1 in, 9 out]
        n58 = Merge Errors(w118, w120) -> (w122:errorcluster)
      }
      frame "Error" {
        w128 = TRUE ("Priority Message? (F)")
        w127 = "Exit" ("Message")
        n59 = Variant To Data(error in=w148, type=errorcluster {"status"=FALSE, "code"=0, "source"=""} ("error out"), Variant=w159) -> (data=w156:errorcluster, error out=w125:errorcluster)
        n60 = call <vilib>:"Simple Error Handler.vi"("error in (no error)"=w156) -> ()  [unwired: 1 in, 8 out]
        n61 = Unbundle By Name(w129) -> ("Message Handler Loop"=w139:refnum<queue>)
        n62 = Unbundle By Name(w129) -> ("Parameter Analyzer"=w154:refnum<queue>)
        n63 = Unbundle By Name(w129) -> ("Switching Matrix"=w149:refnum<queue>)
        n64 = Unbundle By Name(w129) -> ("Optical Spectrometer"=w150:refnum<queue>)
        n65 = Unbundle By Name(w129) -> ("Switches & Mirrors"=w140:refnum<queue>)
        n66 = Unbundle By Name(w129) -> ("Stress Control"=w153:refnum<queue>)
        n67 = Unbundle By Name(w129) -> ("XYZ Stage"=w155:refnum<queue>)
        n68 = Unbundle By Name(w129) -> ("Camera"=w141:refnum<queue>)
        n69 = call "Enqueue Message (Single).vi"("Priority Message? (F)"=w128, "error in (no error)"=w125, "Message"=w127, "Message Queue"=w139) -> ("error out"=w138:errorcluster)  [unwired: 1 in, 6 out]
        n70 = call "Enqueue Message (Single).vi"("Priority Message? (F)"=w128, "error in (no error)"=w125, "Message"=w127, "Message Queue"=w153) -> ("error out"=w147:errorcluster)  [unwired: 1 in, 6 out]
        n71 = call "Enqueue Message (Single).vi"("Priority Message? (F)"=w128, "error in (no error)"=w125, "Message"=w127, "Message Queue"=w154) -> ("error out"=w146:errorcluster)  [unwired: 1 in, 6 out]
        n72 = call "Enqueue Message (Single).vi"("Priority Message? (F)"=w128, "error in (no error)"=w125, "Message"=w127, "Message Queue"=w155) -> ("error out"=w145:errorcluster)  [unwired: 1 in, 6 out]
        n73 = call "Enqueue Message (Single).vi"("Priority Message? (F)"=w128, "error in (no error)"=w125, "Message"=w127, "Message Queue"=w141) -> ("error out"=w144:errorcluster)  [unwired: 1 in, 6 out]
        n74 = call "Enqueue Message (Single).vi"("Priority Message? (F)"=w128, "error in (no error)"=w125, "Message"=w127, "Message Queue"=w140) -> ("error out"=w143:errorcluster)  [unwired: 1 in, 6 out]
        n75 = call "Enqueue Message (Single).vi"("Priority Message? (F)"=w128, "error in (no error)"=w125, "Message"=w127, "Message Queue"=w150) -> ("error out"=w152:errorcluster)  [unwired: 1 in, 6 out]
        n76 = call "Enqueue Message (Single).vi"("Priority Message? (F)"=w128, "error in (no error)"=w125, "Message"=w127, "Message Queue"=w149) -> ("error out"=w151:errorcluster)  [unwired: 1 in, 6 out]
        n77 = Merge Errors(w138, w147, w146, w145, w144, w143, w152, w151) -> (w142:errorcluster)
        n78 = Unbundle By Name(w129) -> ("Instrument Sequence"=w135:refnum<queue>)
        n79 = Unbundle By Name(w129) -> ("Strain Measurement"=w131:refnum<queue>)
        n80 = Unbundle By Name(w129) -> ("AutoFocus"=w137:refnum<queue>)
        n81 = Unbundle By Name(w129) -> ("Save Data"=w136:refnum<queue>)
        n82 = Unbundle By Name(w129) -> ("Plot Data"=w124:refnum<queue>)
        n83 = call "Enqueue Message (Single).vi"("Priority Message? (F)"=w128, "error in (no error)"=w125, "Message"=w127, "Message Queue"=w137) -> ("error out"=w132:errorcluster)  [unwired: 1 in, 6 out]
        n84 = call "Enqueue Message (Single).vi"("Priority Message? (F)"=w128, "error in (no error)"=w125, "Message"=w127, "Message Queue"=w136) -> ("error out"=w133:errorcluster)  [unwired: 1 in, 6 out]
        n85 = call "Enqueue Message (Single).vi"("Priority Message? (F)"=w128, "error in (no error)"=w125, "Message"=w127, "Message Queue"=w135) -> ("error out"=w134:errorcluster)  [unwired: 1 in, 6 out]
        n86 = call "Enqueue Message (Single).vi"("Priority Message? (F)"=w128, "error in (no error)"=w125, "Message"=w127, "Message Queue"=w131) -> ("error out"=w130:errorcluster)  [unwired: 1 in, 6 out]
        n87 = call "Enqueue Message (Single).vi"("Priority Message? (F)"=w128, "error in (no error)"=w125, "Message"=w127, "Message Queue"=w124) -> ("error out"=w126:errorcluster)  [unwired: 1 in, 6 out]
        n88 = Merge Errors(w132, w133, w134, w130, w126) -> (w123:errorcluster)
        n89 = Merge Errors(w123, w142) -> (w157:errorcluster)
      }
      frame "----- Other UI Events -----" {
        # "Other UI Events"
      }
      frame "Other UI - Update Status" {
        n90 = Variant To Data(error in=w168, type="", Variant=w167) -> (data=w161:string, error out=w165:errorcluster)
        "Last Operation" <- w161
        n91 = call "Status String.vi"("Message"=w161) -> ("Status String"=w164:string)
        n92 = property on="Status Log" class="Str"() -> ("Value"=w162:string)  [unwired: 2 in, 2 out]
        n93 = Concatenate Strings(w164, w162) -> (→"Status Log":string)
      }
      frame "----- Labram HR Events -----" {
        # "Labram HR Events"
      }
      frame "LabramHR - Set Laser" {
        # "Handle the change of Excitation Wavelength"
        n94 = Variant To Data(error in=w176, type=Laser."633 nm" ("NewVal"), Variant=w180) -> (data=w171:T29, error out=w175:errorcluster)
        n95 = Bundle By Name(cluster=T27 {"Laser Settings"={"Laser Wavelength"=enum."633 nm", "Neutral Density Filter"=enum."1%"}, "Spectrometer Settings"={"Confocal Hole Size (µm)"=150.0, "Grating"=1, "Detector"=enum."InGaAs Array"}, "Acquisition Settings"={"Acquisition Mode"=enum."Single Window", "Spectal Position (nm)"=480.0, "From (nm)"=632.0, "To (nm)"=1000.0, "Integration Time (s)"=3.0, "Number of Accumulations"=3, "AutoScanning"=FALSE, "Spike Removal"=FALSE}, "Path"=path ""} ("LabramHR"), "Laser Settings.Laser Wavelength"=w171) -> (w173:T27)
        n96 = Unbundle By Name(w179) -> ("Optical Spectrometer"=w178:refnum<queue>)
        n97 = call "Enqueue Message (Single).vi"("error in (no error)"=w175, "Message Data"=w173, "Message"="Set Laser", "Message Queue"=w178) -> ("error out"=w174:errorcluster)  [unwired: 7 out]
      }
      frame "LabramHR - Set Filter" {
        # "Handle the change of Neutral Density Filter"
        n98 = Variant To Data(error in=w191, type=Filter."1%" ("NewVal"), Variant=w190) -> (data=w182:T30, error out=w188:errorcluster)
        n99 = Bundle By Name(cluster=T27 {"Laser Settings"={"Laser Wavelength"=enum."633 nm", "Neutral Density Filter"=enum."1%"}, "Spectrometer Settings"={"Confocal Hole Size (µm)"=150.0, "Grating"=1, "Detector"=enum."InGaAs Array"}, "Acquisition Settings"={"Acquisition Mode"=enum."Single Window", "Spectal Position (nm)"=480.0, "From (nm)"=632.0, "To (nm)"=1000.0, "Integration Time (s)"=3.0, "Number of Accumulations"=3, "AutoScanning"=FALSE, "Spike Removal"=FALSE}, "Path"=path ""} ("LabramHR"), "Laser Settings.Neutral Density Filter"=w182) -> (w184:T27)
        n100 = Unbundle By Name(w186) -> ("Optical Spectrometer"=w189:refnum<queue>)
        n101 = call "Enqueue Message (Single).vi"("error in (no error)"=w188, "Message Data"=w184, "Message"="Set Filter", "Message Queue"=w189) -> ("error out"=w187:errorcluster)  [unwired: 7 out]
      }
      frame "LabramHR - Set Hole" {
        # "Handle the change in Confocal hole size"
        n102 = Variant To Data(error in=w202, type=150.0 ("Confocal Hole Size (µm) 2"), Variant=w201) -> (data=w194:dbl, error out=w197:errorcluster)
        n103 = Bundle By Name(cluster=T27 {"Laser Settings"={"Laser Wavelength"=enum."633 nm", "Neutral Density Filter"=enum."1%"}, "Spectrometer Settings"={"Confocal Hole Size (µm)"=150.0, "Grating"=1, "Detector"=enum."InGaAs Array"}, "Acquisition Settings"={"Acquisition Mode"=enum."Single Window", "Spectal Position (nm)"=480.0, "From (nm)"=632.0, "To (nm)"=1000.0, "Integration Time (s)"=3.0, "Number of Accumulations"=3, "AutoScanning"=FALSE, "Spike Removal"=FALSE}, "Path"=path ""} ("LabramHR"), "Spectrometer Settings.Confocal Hole Size (µm)"=w194) -> (w193:T27)
        n104 = Unbundle By Name(w195) -> ("Optical Spectrometer"=w199:refnum<queue>)
        n105 = call "Enqueue Message (Single).vi"("error in (no error)"=w197, "Message Data"=w193, "Message"="Set Hole", "Message Queue"=w199) -> ("error out"=w198:errorcluster)  [unwired: 7 out]
      }
      frame "LabramHR - Set Grating" {
        w204 = T32 1 items=["1800 l/mm", "150 l/mm"] ("NewVal")
        # "Handle the change of grating"
        n106 = Variant To Data(error in=w213, type=w204, Variant=w212) -> (data=w206:T32, error out=w209:errorcluster)
        n107 = Bundle By Name(cluster=T27 {"Laser Settings"={"Laser Wavelength"=enum."633 nm", "Neutral Density Filter"=enum."1%"}, "Spectrometer Settings"={"Confocal Hole Size (µm)"=150.0, "Grating"=1, "Detector"=enum."InGaAs Array"}, "Acquisition Settings"={"Acquisition Mode"=enum."Single Window", "Spectal Position (nm)"=480.0, "From (nm)"=632.0, "To (nm)"=1000.0, "Integration Time (s)"=3.0, "Number of Accumulations"=3, "AutoScanning"=FALSE, "Spike Removal"=FALSE}, "Path"=path ""} ("LabramHR"), "Spectrometer Settings.Grating"=w206) -> (w205:T27)
        n108 = Unbundle By Name(w208) -> ("Optical Spectrometer"=w211:refnum<queue>)
        n109 = call "Enqueue Message (Single).vi"("error in (no error)"=w209, "Message Data"=w205, "Message"="Set Grating", "Message Queue"=w211) -> ("error out"=w210:errorcluster)  [unwired: 7 out]
      }
      frame "LabramHR - Set Detector" {
        # "Handle the change of grating"
        n110 = Variant To Data(error in=w224, type=Detector."Silicon CCD" ("NewVal"), Variant=w223) -> (data=w217:T33, error out=w220:errorcluster)
        n111 = Bundle By Name(cluster=T27 {"Laser Settings"={"Laser Wavelength"=enum."633 nm", "Neutral Density Filter"=enum."1%"}, "Spectrometer Settings"={"Confocal Hole Size (µm)"=150.0, "Grating"=1, "Detector"=enum."InGaAs Array"}, "Acquisition Settings"={"Acquisition Mode"=enum."Single Window", "Spectal Position (nm)"=480.0, "From (nm)"=632.0, "To (nm)"=1000.0, "Integration Time (s)"=3.0, "Number of Accumulations"=3, "AutoScanning"=FALSE, "Spike Removal"=FALSE}, "Path"=path ""} ("LabramHR"), "Spectrometer Settings.Detector"=w217) -> (w216:T27)
        n112 = Unbundle By Name(w219) -> ("Optical Spectrometer"=w222:refnum<queue>)
        n113 = call "Enqueue Message (Single).vi"("error in (no error)"=w220, "Message Data"=w216, "Message"="Set Detector", "Message Queue"=w222) -> ("error out"=w221:errorcluster)  [unwired: 7 out]
      }
      frame "LabramHR - Set Spectal Position" {
        # "Handle the change of Spetrometer position"
        n114 = Variant To Data(error in=w235, type=480.0 ("Spectal Position (nm) 2"), Variant=w234) -> (data=w227:dbl, error out=w229:errorcluster)
        n115 = Bundle By Name(cluster=T27 {"Laser Settings"={"Laser Wavelength"=enum."633 nm", "Neutral Density Filter"=enum."1%"}, "Spectrometer Settings"={"Confocal Hole Size (µm)"=150.0, "Grating"=1, "Detector"=enum."InGaAs Array"}, "Acquisition Settings"={"Acquisition Mode"=enum."Single Window", "Spectal Position (nm)"=480.0, "From (nm)"=632.0, "To (nm)"=1000.0, "Integration Time (s)"=3.0, "Number of Accumulations"=3, "AutoScanning"=FALSE, "Spike Removal"=FALSE}, "Path"=path ""} ("LabramHR"), "Acquisition Settings.Spectal Position (nm)"=w227) -> (w226:T27)
        n116 = Unbundle By Name(w228) -> ("Optical Spectrometer"=w232:refnum<queue>)
        n117 = call "Enqueue Message (Single).vi"("error in (no error)"=w229, "Message Data"=w226, "Message"="Set Spectal Position", "Message Queue"=w232) -> ("error out"=w231:errorcluster)  [unwired: 7 out]
      }
      frame "LabramHR - Set Acquisition Settings" {
        # "Handle the change of integration time"
        n118 = Variant To Data(error in=w246, type=T34 {"Acquisition Mode"=enum."Single Window", "Spectal Position (nm)"=480.0, "From (nm)"=632.0, "To (nm)"=1000.0, "Integration Time (s)"=3.0, "Number of Accumulations"=3, "AutoScanning"=FALSE, "Spike Removal"=FALSE} ("Acquisition Settings 2"), Variant=w245) -> (data=w239:T34, error out=w243:errorcluster)
        n119 = Bundle By Name(cluster=T27 {"Laser Settings"={"Laser Wavelength"=enum."633 nm", "Neutral Density Filter"=enum."1%"}, "Spectrometer Settings"={"Confocal Hole Size (µm)"=150.0, "Grating"=1, "Detector"=enum."InGaAs Array"}, "Acquisition Settings"={"Acquisition Mode"=enum."Single Window", "Spectal Position (nm)"=480.0, "From (nm)"=632.0, "To (nm)"=1000.0, "Integration Time (s)"=3.0, "Number of Accumulations"=3, "AutoScanning"=FALSE, "Spike Removal"=FALSE}, "Path"=path ""} ("LabramHR"), "Acquisition Settings"=w239) -> (w238:T27)
        n120 = Unbundle By Name(w240) -> ("Optical Spectrometer"=w241:refnum<queue>)
        n121 = call "Enqueue Message (Single).vi"("error in (no error)"=w243, "Message Data"=w238, "Message"="Set Acquisition Settings", "Message Queue"=w241) -> ("error out"=w244:errorcluster)  [unwired: 7 out]
      }
      frame "LabramHR - Acquire Spectrum" {
        n122 = Unbundle By Name(w248) -> ("Optical Spectrometer"=w249:refnum<queue>)
        n123 = call "Enqueue Message (Single).vi"("error in (no error)"=w250, "Message"="Acquire Spectrum", "Message Queue"=w249) -> ("error out"=w247:errorcluster)  [unwired: 1 in, 7 out]
      }
      frame "LabramHR - Save Spectrum" {
        n124 = Unbundle By Name(w253) -> ("Optical Spectrometer"=w254:refnum<queue>)
        n125 = call "Enqueue Message (Single).vi"("error in (no error)"=w255, "Message"="Save Optical Spectrum", "Message Queue"=w254) -> ("error out"=w252:errorcluster)  [unwired: 1 in, 7 out]
      }
      frame "----- Switches & Mirrors Events -----" {
        # "Switches & Mirrors EVENTS"
      }
      frame "Switches & Mirrors - Set UI" {
        n126 = Variant To Data(error in=w265, type=T35 {"Relay VISA Session"="COM1", "Switches"={"Laser"=FALSE, "Video"=FALSE}, "Delays (ms)"={"Laser"=500, "Video"=1500}} ("Laser-Video Config"), Variant=w260) -> (data=w259:T35, error out=w261:errorcluster)
        n127 = Unbundle By Name(w259) -> ("Switches.Laser"=w264:bool, "Switches.Video"=w263:bool, "Relay VISA Session"=w262:refnum<visa-resource-name>)
        n128 = property on="Video" class="Bool (strict)"("Value"=w264) -> ()  [unwired: 2 in, 2 out]
        n129 = property on="Laser" class="Bool (strict)"("Value"=w263) -> ()  [unwired: 2 in, 2 out]
        n130 = property on="Switches & Mirrors VISA Session" class="VISAName"("Value"=w262) -> ()  [unwired: 2 in, 2 out]
      }
      frame "Switches & Mirrors - Update Refnums" {
        n131 = control-ref of="Switches & Mirrors VISA Session"() -> (w272:refnum<vi>)
        n132 = control-ref of="Laser"() -> (w273:refnum<vi>)
        n133 = control-ref of="Video"() -> (w271:refnum<vi>)
        n134 = control-ref of="Instrument Status"() -> (w266:refnum<vi>)
        n135 = Bundle By Name(cluster=T59 {"Instrument Status"=refnum, "Laser"=refnum, "Video"=refnum, "Relay VISA"=refnum} ("Laser Video Refnums"), "Instrument Status"=w266, "Laser"=w273, "Video"=w271, "Relay VISA"=w272) -> (w268:T59)
        n136 = Unbundle By Name(w274) -> ("Switches & Mirrors"=w275:refnum<queue>)
        n137 = call "Enqueue Message (Single).vi"("error in (no error)"=w270, "Message Data"=w268, "Message"="Update Refnums", "Message Queue"=w275) -> ("error out"=w276:errorcluster)  [unwired: 7 out]
      }
      frame "Switches & Mirrors - Update Visa Session" {
        n138 = Variant To Data(error in=w284, type=refnum<visa-resource-name> "COM1" ("Laser Video VISA Session 2"), Variant=w280) -> (data=w279:refnum<visa-resource-name>, error out=w282:errorcluster)
        n139 = Bundle By Name(cluster=T35 {"Relay VISA Session"="COM1", "Switches"={"Laser"=FALSE, "Video"=FALSE}, "Delays (ms)"={"Laser"=500, "Video"=1500}} ("Laser-Video Config"), "Relay VISA Session"=w279) -> (w278:T35)
        n140 = Unbundle By Name(w285) -> ("Switches & Mirrors"=w286:refnum<queue>)
        n141 = call "Enqueue Message (Single).vi"("error in (no error)"=w282, "Message Data"=w278, "Message"="Update VISA Session", "Message Queue"=w286) -> ("error out"=w287:errorcluster)  [unwired: 7 out]
      }
      frame "Switches & Mirrors - Update Laser" {
        n142 = Variant To Data(error in=w297, type=FALSE ("Laser"), Variant=w298) -> (data=w288:bool, error out=w295:errorcluster)
        n143 = Bundle By Name(cluster=T35 {"Relay VISA Session"="COM1", "Switches"={"Laser"=FALSE, "Video"=FALSE}, "Delays (ms)"={"Laser"=500, "Video"=1500}} ("Laser-Video Config"), "Switches.Laser"=w288) -> (w291:T35)
        n144 = Unbundle By Name(w293) -> ("Switches & Mirrors"=w294:refnum<queue>)
        n145 = call "Enqueue Message (Single).vi"("error in (no error)"=w295, "Message Data"=w291, "Message"="Update Laser", "Message Queue"=w294) -> ("error out"=w296:errorcluster)  [unwired: 7 out]
      }
      frame "Switches & Mirrors - Update Video" {
        n146 = Variant To Data(error in=w308, type=FALSE ("Laser"), Variant=w309) -> (data=w299:bool, error out=w306:errorcluster)
        n147 = Bundle By Name(cluster=T35 {"Relay VISA Session"="COM1", "Switches"={"Laser"=FALSE, "Video"=FALSE}, "Delays (ms)"={"Laser"=500, "Video"=1500}} ("Laser-Video Config"), "Switches.Video"=w299) -> (w302:T35)
        n148 = Unbundle By Name(w304) -> ("Switches & Mirrors"=w305:refnum<queue>)
        n149 = call "Enqueue Message (Single).vi"("error in (no error)"=w306, "Message Data"=w302, "Message"="Update Video", "Message Queue"=w305) -> ("error out"=w307:errorcluster)  [unwired: 7 out]
      }
      frame "----- Camera Events -----" {
        # "uEye Camera EVENTS"
      }
      frame "Camera - Update Settings" {
        w313 = T37 {"Settings"={"Pixel clock"=20, "Frame rate"=30.0, "Exposure time"=33.21525, "Master Gain"=0, "Red Gain"=0, "Green Gain"=0, "Blue Gain"=0, "Auto Gain"=FALSE, "White-balance"=FALSE, "Color Correction"=FALSE}} ("Camera Configuration")
        n150 = Unbundle By Name(w313) -> ("Settings"=w314:T38)
        n151 = Variant To Data(error in=w320, type=w314, Variant=w321) -> (data=w311:T38, error out=w315:errorcluster)
        n152 = Bundle By Name(cluster=w313, "Settings"=w311) -> (w312:T37)
        n153 = Unbundle By Name(w317) -> ("Camera"=w318:refnum<queue>)
        n154 = call "Enqueue Message (Single).vi"("error in (no error)"=w315, "Message Data"=w312, "Message"="Update Settings", "Message Queue"=w318) -> ("error out"=w319:errorcluster)  [unwired: 7 out]
      }
      frame "Camera - Start Live" {
        n155 = Unbundle By Name(w324) -> ("Camera"=w325:refnum<queue>)
        n156 = call "Enqueue Message (Single).vi"("error in (no error)"=w322, "Message"="Start Live", "Message Queue"=w325) -> ("error out"=w326:errorcluster)  [unwired: 1 in, 7 out]
      }
      frame "Camera - Stop Live" {
        n157 = Unbundle By Name(w329) -> ("Camera"=w330:refnum<queue>)
        n158 = call "Enqueue Message (Single).vi"("error in (no error)"=w327, "Message"="Stop Live", "Message Queue"=w330) -> ("error out"=w331:errorcluster)  [unwired: 1 in, 7 out]
      }
      frame "----- Stress Control Events -----" {
        # "Stress Control Events"
      }
      frame "Stress Control - Update Motion Mode" {
        w336 = u16 0 items=["Absolute", "Relative"] ("Motion 2")
        n159 = Variant To Data(error in=w343, type=w336, Variant=w337) -> (data=w335:u16, error out=w338:errorcluster)
        n160 = Bundle By Name(cluster=T26 {"Stress Control VISA Session"="", "Axis"=1, "Motion"=0, "Destination (°)"=0.0, "Speed (°/s)"=4.0, "Position (°)"=0.0} ("Stress Control Configuration"), "Motion"=w335) -> (w334:T26)
        n161 = Unbundle By Name(w339) -> ("Stress Control"=w340:refnum<queue>)
        n162 = call "Enqueue Message (Single).vi"("error in (no error)"=w338, "Message Data"=w334, "Message"="Update Motion Mode", "Message Queue"=w340) -> ("error out"=w342:errorcluster)  [unwired: 7 out]
      }
      frame "Stress Control - Update Destination" {
        n163 = Variant To Data(error in=w354, type=0.0 ("Destination (°) 2"), Variant=w348) -> (data=w347:dbl, error out=w349:errorcluster)
        n164 = Bundle By Name(cluster=T26 {"Stress Control VISA Session"="", "Axis"=1, "Motion"=0, "Destination (°)"=0.0, "Speed (°/s)"=4.0, "Position (°)"=0.0} ("Stress Control Configuration"), "Destination (°)"=w347) -> (w345:T26)
        n165 = Unbundle By Name(w350) -> ("Stress Control"=w351:refnum<queue>)
        n166 = call "Enqueue Message (Single).vi"("error in (no error)"=w349, "Message Data"=w345, "Message"="Update Destination", "Message Queue"=w351) -> ("error out"=w353:errorcluster)  [unwired: 7 out]
      }
      frame "Stress Control - Change Stress" {
        n167 = Unbundle By Name(w357) -> ("Stress Control"=w358:refnum<queue>)
        n168 = call "Enqueue Message (Single).vi"("error in (no error)"=w355, "Message"="Change Stress", "Message Queue"=w358) -> ("error out"=w359:errorcluster)  [unwired: 1 in, 7 out]
      }
      frame "----- Parameter Analyzer Events -----" {
        # "Parameter Analyzer Events"
      }
      frame "Parameter Analyzer - Set Settings" {
        n169 = Variant To Data(error in=w364, type=T17 {"Parameter Analyzer VISA Session"="COM1", "Sweeping Time Parameters"={"Integration Time"=0, "Short Integration Time (s)"=0.0, "Long Integration Time (s)"=0.0, "Wait Time Parameter"=1.0}, "Acquisition Mode"=enum."Sweeping Mode", "Status Polling Time (ms)"=1000, "Comment"="Test VI", "SMU 1 - Sweeping"={"Start / Offset"=0.0, "Stop / Ratio"=1.0, "Step \n(linear only)"=0.01, "Compliance"=0.1, "Power \nCompliance"=0.0, "Mode"=0, "Function"=0, "Sweep Mode"=FALSE}, "SMU 2 - Sweeping"={"Start / Offset"=0.0, "Stop / Ratio"=1.0, "Step \n(linear only)"=0.01, "Compliance"=0.1, "Power \nCompliance"=0.0, "Mode"=0, "Function"=0, "Sweep Mode"=FALSE}, "SMU 3 - Sweeping"={"Start / Offset"=0.0, "Stop / Ratio"=1.0, "Step \n(linear only)"=0.01, "Compliance"=0.1, "Power \nCompliance"=0.0, "Mode"=0, "Function"=0, "Sweep Mode"=FALSE}, "SMU 4 - Sweeping"={"Start / Offset"=0.0, "Stop / Ratio"=1.0, "Step \n(linear only)"=0.01, "Compliance"=0.1, "Power \nCompliance"=0.0, "Mode"=1, "Function"=0, "Sweep Mode"=FALSE}, "Sweep Spacing"=0, "Range"=0, "SMU1 - Sampling"={"Source"=10.0, "Compliance"=1e-05, "Mode"=0, "Function"=FALSE}, "SMU2 - Sampling"={"Source"=10.0, "Compliance"=1e-05, "Mode"=0, "Function"=FALSE}, "SMU3 - Sampling"={"Source"=10.0, "Compliance"=1e-05, "Mode"=0, "Function"=FALSE}, "SMU4 - Sampling"={"Source"=10.0, "Compliance"=1e-05, "Mode"=0, "Function"=FALSE}, "Sampling Time Parameters"={"Initial Interval (s)"=0.1, "Number of Samples"=60, "Total Sampling Time (s)"=10.0, "Hold Time (s)"=0.0, "Sampling Mode"=0, "Sampling Time"=0}, "Stop Condition"={"Enable Delay (s)"=0.0, "Name"="", "Threshold"=0.0, "num. of events"=1, "Event"=0, "Stop Condition Enable"=FALSE}} ("HP4155C Configuration"), Variant=w362) -> (error out=w363:errorcluster)  [unwired: 1 out]
      }
      frame "Parameter Analyzer - Update Visa Session" {
        w366 = T17 {"Parameter Analyzer VISA Session"="COM1", "Sweeping Time Parameters"={"Integration Time"=0, "Short Integration Time (s)"=0.0, "Long Integration Time (s)"=0.0, "Wait Time Parameter"=1.0}, "Acquisition Mode"=enum."Sweeping Mode", "Status Polling Time (ms)"=1000, "Comment"="Test VI", "SMU 1 - Sweeping"={"Start / Offset"=0.0, "Stop / Ratio"=1.0, "Step \n(linear only)"=0.01, "Compliance"=0.1, "Power \nCompliance"=0.0, "Mode"=0, "Function"=0, "Sweep Mode"=FALSE}, "SMU 2 - Sweeping"={"Start / Offset"=0.0, "Stop / Ratio"=1.0, "Step \n(linear only)"=0.01, "Compliance"=0.1, "Power \nCompliance"=0.0, "Mode"=0, "Function"=0, "Sweep Mode"=FALSE}, "SMU 3 - Sweeping"={"Start / Offset"=0.0, "Stop / Ratio"=1.0, "Step \n(linear only)"=0.01, "Compliance"=0.1, "Power \nCompliance"=0.0, "Mode"=0, "Function"=0, "Sweep Mode"=FALSE}, "SMU 4 - Sweeping"={"Start / Offset"=0.0, "Stop / Ratio"=1.0, "Step \n(linear only)"=0.01, "Compliance"=0.1, "Power \nCompliance"=0.0, "Mode"=1, "Function"=0, "Sweep Mode"=FALSE}, "Sweep Spacing"=0, "Range"=0, "SMU1 - Sampling"={"Source"=10.0, "Compliance"=1e-05, "Mode"=0, "Function"=FALSE}, "SMU2 - Sampling"={"Source"=10.0, "Compliance"=1e-05, "Mode"=0, "Function"=FALSE}, "SMU3 - Sampling"={"Source"=10.0, "Compliance"=1e-05, "Mode"=0, "Function"=FALSE}, "SMU4 - Sampling"={"Source"=10.0, "Compliance"=1e-05, "Mode"=0, "Function"=FALSE}, "Sampling Time Parameters"={"Initial Interval (s)"=0.1, "Number of Samples"=60, "Total Sampling Time (s)"=10.0, "Hold Time (s)"=0.0, "Sampling Mode"=0, "Sampling Time"=0}, "Stop Condition"={"Enable Delay (s)"=0.0, "Name"="", "Threshold"=0.0, "num. of events"=1, "Event"=0, "Stop Condition Enable"=FALSE}} ("HP4155C Configuration")
        n170 = Unbundle By Name(w366) -> ("Parameter Analyzer VISA Session"=w367:refnum<visa-resource-name>)
        n171 = Variant To Data(error in=w375, type=w367, Variant=w374) -> (data=w365:refnum<visa-resource-name>, error out=w370:errorcluster)
        n172 = Bundle By Name(cluster=w366, "Parameter Analyzer VISA Session"=w365) -> (w368:T17)
        n173 = Unbundle By Name(w371) -> ("Parameter Analyzer"=w372:refnum<queue>)
        n174 = call "Enqueue Message (Single).vi"("error in (no error)"=w370, "Message Data"=w368, "Message"="Update Visa Session", "Message Queue"=w372) -> ("error out"=w369:errorcluster)  [unwired: 7 out]
      }
      frame "Parameter Analyzer - Configure Integration time" {
        w376 = T17 {"Parameter Analyzer VISA Session"="COM1", "Sweeping Time Parameters"={"Integration Time"=0, "Short Integration Time (s)"=0.0, "Long Integration Time (s)"=0.0, "Wait Time Parameter"=1.0}, "Acquisition Mode"=enum."Sweeping Mode", "Status Polling Time (ms)"=1000, "Comment"="Test VI", "SMU 1 - Sweeping"={"Start / Offset"=0.0, "Stop / Ratio"=1.0, "Step \n(linear only)"=0.01, "Compliance"=0.1, "Power \nCompliance"=0.0, "Mode"=0, "Function"=0, "Sweep Mode"=FALSE}, "SMU 2 - Sweeping"={"Start / Offset"=0.0, "Stop / Ratio"=1.0, "Step \n(linear only)"=0.01, "Compliance"=0.1, "Power \nCompliance"=0.0, "Mode"=0, "Function"=0, "Sweep Mode"=FALSE}, "SMU 3 - Sweeping"={"Start / Offset"=0.0, "Stop / Ratio"=1.0, "Step \n(linear only)"=0.01, "Compliance"=0.1, "Power \nCompliance"=0.0, "Mode"=0, "Function"=0, "Sweep Mode"=FALSE}, "SMU 4 - Sweeping"={"Start / Offset"=0.0, "Stop / Ratio"=1.0, "Step \n(linear only)"=0.01, "Compliance"=0.1, "Power \nCompliance"=0.0, "Mode"=1, "Function"=0, "Sweep Mode"=FALSE}, "Sweep Spacing"=0, "Range"=0, "SMU1 - Sampling"={"Source"=10.0, "Compliance"=1e-05, "Mode"=0, "Function"=FALSE}, "SMU2 - Sampling"={"Source"=10.0, "Compliance"=1e-05, "Mode"=0, "Function"=FALSE}, "SMU3 - Sampling"={"Source"=10.0, "Compliance"=1e-05, "Mode"=0, "Function"=FALSE}, "SMU4 - Sampling"={"Source"=10.0, "Compliance"=1e-05, "Mode"=0, "Function"=FALSE}, "Sampling Time Parameters"={"Initial Interval (s)"=0.1, "Number of Samples"=60, "Total Sampling Time (s)"=10.0, "Hold Time (s)"=0.0, "Sampling Mode"=0, "Sampling Time"=0}, "Stop Condition"={"Enable Delay (s)"=0.0, "Name"="", "Threshold"=0.0, "num. of events"=1, "Event"=0, "Stop Condition Enable"=FALSE}} ("HP4155C Configuration")
        n175 = Unbundle By Name(w376) -> ("Sweeping Time Parameters"=w377:T18)
        n176 = Variant To Data(error in=w386, type=w377, Variant=w385) -> (data=w378:T18, error out=w382:errorcluster)
        n177 = Bundle By Name(cluster=w376, "Sweeping Time Parameters"=w378) -> (w379:T17)
        n178 = Unbundle By Name(w380) -> ("Parameter Analyzer"=w383:refnum<queue>)
        n179 = call "Enqueue Message (Single).vi"("error in (no error)"=w382, "Message Data"=w379, "Message"="Configure Integration Time", "Message Queue"=w383) -> ("error out"=w381:errorcluster)  [unwired: 7 out]
      }
      frame "Parameter Analyzer - Configure Sweeping" {
        n180 = Variant To Data(error in=w403, type=T60 {"SMU 1 - Sweeping"={"Start / Offset"=0.0, "Stop / Ratio"=0.0, "Step (linear only)"=0.0, "Compliance"=0.0, "Power Compliance"=0.0, "Mode"=0, "Function"=0, "Sweep Mode"=FALSE}, "SMU 2 - Sweeping"={"Start / Offset"=0.0, "Stop / Ratio"=0.0, "Step (linear only)"=0.0, "Compliance"=0.0, "Power Compliance"=0.0, "Mode"=0, "Function"=0, "Sweep Mode"=FALSE}, "SMU 3 - Sweeping"={"Start / Offset"=0.0, "Stop / Ratio"=0.0, "Step (linear only)"=0.0, "Compliance"=0.0, "Power Compliance"=0.0, "Mode"=0, "Function"=0, "Sweep Mode"=FALSE}, "SMU 4 - Sweeping"={"Start / Offset"=0.0, "Stop / Ratio"=0.0, "Step (linear only)"=0.0, "Compliance"=0.0, "Power Compliance"=0.0, "Mode"=0, "Function"=0, "Sweep Mode"=FALSE}, "Sweep Spacing"=0, "Range"=0} ("output cluster"), Variant=w402) -> (data=w401:T60, error out=w393:errorcluster)
        n181 = Unbundle By Name(w401) -> ("SMU 1 - Sweeping"=w396:T63, "SMU 2 - Sweeping"=w397:T63, "SMU 3 - Sweeping"=w398:T63, "SMU 4 - Sweeping"=w399:T63, "Sweep Spacing"=w400:u16, "Range"=w390:u16)
        n182 = Bundle By Name(cluster=T17 {"Parameter Analyzer VISA Session"="COM1", "Sweeping Time Parameters"={"Integration Time"=0, "Short Integration Time (s)"=0.0, "Long Integration Time (s)"=0.0, "Wait Time Parameter"=1.0}, "Acquisition Mode"=enum."Sweeping Mode", "Status Polling Time (ms)"=1000, "Comment"="Test VI", "SMU 1 - Sweeping"={"Start / Offset"=0.0, "Stop / Ratio"=1.0, "Step \n(linear only)"=0.01, "Compliance"=0.1, "Power \nCompliance"=0.0, "Mode"=0, "Function"=0, "Sweep Mode"=FALSE}, "SMU 2 - Sweeping"={"Start / Offset"=0.0, "Stop / Ratio"=1.0, "Step \n(linear only)"=0.01, "Compliance"=0.1, "Power \nCompliance"=0.0, "Mode"=0, "Function"=0, "Sweep Mode"=FALSE}, "SMU 3 - Sweeping"={"Start / Offset"=0.0, "Stop / Ratio"=1.0, "Step \n(linear only)"=0.01, "Compliance"=0.1, "Power \nCompliance"=0.0, "Mode"=0, "Function"=0, "Sweep Mode"=FALSE}, "SMU 4 - Sweeping"={"Start / Offset"=0.0, "Stop / Ratio"=1.0, "Step \n(linear only)"=0.01, "Compliance"=0.1, "Power \nCompliance"=0.0, "Mode"=1, "Function"=0, "Sweep Mode"=FALSE}, "Sweep Spacing"=0, "Range"=0, "SMU1 - Sampling"={"Source"=10.0, "Compliance"=1e-05, "Mode"=0, "Function"=FALSE}, "SMU2 - Sampling"={"Source"=10.0, "Compliance"=1e-05, "Mode"=0, "Function"=FALSE}, "SMU3 - Sampling"={"Source"=10.0, "Compliance"=1e-05, "Mode"=0, "Function"=FALSE}, "SMU4 - Sampling"={"Source"=10.0, "Compliance"=1e-05, "Mode"=0, "Function"=FALSE}, "Sampling Time Parameters"={"Initial Interval (s)"=0.1, "Number of Samples"=60, "Total Sampling Time (s)"=10.0, "Hold Time (s)"=0.0, "Sampling Mode"=0, "Sampling Time"=0}, "Stop Condition"={"Enable Delay (s)"=0.0, "Name"="", "Threshold"=0.0, "num. of events"=1, "Event"=0, "Stop Condition Enable"=FALSE}} ("HP4155C Configuration"), "SMU 1 - Sweeping"=w396, "SMU 2 - Sweeping"=w397, "SMU 3 - Sweeping"=w398, "SMU 4 - Sweeping"=w399, "Sweep Spacing"=w400, "Range"=w390) -> (w389:T17)
        n183 = Unbundle By Name(w391) -> ("Parameter Analyzer"=w394:refnum<queue>)
        n184 = call "Enqueue Message (Single).vi"("error in (no error)"=w393, "Message Data"=w389, "Message"="Configure Sweeping", "Message Queue"=w394) -> ("error out"=w392:errorcluster)  [unwired: 7 out]
      }
      frame "Parameter Analyzer - Configure Sampling" {
        n185 = Variant To Data(error in=w420, type=T61 {"SMU1 - Sampling"={"Source"=0.0, "Compliance"=0.0, "Mode"=0, "Function"=FALSE}, "SMU2 - Sampling"={"Source"=0.0, "Compliance"=0.0, "Mode"=0, "Function"=FALSE}, "SMU3 - Sampling"={"Source"=0.0, "Compliance"=0.0, "Mode"=0, "Function"=FALSE}, "SMU4 - Sampling"={"Source"=0.0, "Compliance"=0.0, "Mode"=0, "Function"=FALSE}, "Sampling Parameters"={"Initial Interval (s)"=0.0, "Number of Samples"=0, "Total Sampling Time (s)"=0.0, "Hold Time (s)"=0.0, "Sampling Mode"=0, "Sampling Time"=0}, "Stop Condition"={"Enable Delay (s)"=0.0, "Name"="", "Threshold"=0.0, "num. of events"=0, "Event"=0, "Stop Condition Enable"=FALSE}} ("output cluster"), Variant=w419) -> (data=w418:T61, error out=w413:errorcluster)
        n186 = Unbundle By Name(w418) -> ("SMU1 - Sampling"=w409:T64, "SMU2 - Sampling"=w408:T64, "SMU3 - Sampling"=w407:T64, "SMU4 - Sampling"=w406:T64, "Sampling Parameters"=w417:T65, "Stop Condition"=w416:T66)
        n187 = Bundle By Name(cluster=T17 {"Parameter Analyzer VISA Session"="COM1", "Sweeping Time Parameters"={"Integration Time"=0, "Short Integration Time (s)"=0.0, "Long Integration Time (s)"=0.0, "Wait Time Parameter"=1.0}, "Acquisition Mode"=enum."Sweeping Mode", "Status Polling Time (ms)"=1000, "Comment"="Test VI", "SMU 1 - Sweeping"={"Start / Offset"=0.0, "Stop / Ratio"=1.0, "Step \n(linear only)"=0.01, "Compliance"=0.1, "Power \nCompliance"=0.0, "Mode"=0, "Function"=0, "Sweep Mode"=FALSE}, "SMU 2 - Sweeping"={"Start / Offset"=0.0, "Stop / Ratio"=1.0, "Step \n(linear only)"=0.01, "Compliance"=0.1, "Power \nCompliance"=0.0, "Mode"=0, "Function"=0, "Sweep Mode"=FALSE}, "SMU 3 - Sweeping"={"Start / Offset"=0.0, "Stop / Ratio"=1.0, "Step \n(linear only)"=0.01, "Compliance"=0.1, "Power \nCompliance"=0.0, "Mode"=0, "Function"=0, "Sweep Mode"=FALSE}, "SMU 4 - Sweeping"={"Start / Offset"=0.0, "Stop / Ratio"=1.0, "Step \n(linear only)"=0.01, "Compliance"=0.1, "Power \nCompliance"=0.0, "Mode"=1, "Function"=0, "Sweep Mode"=FALSE}, "Sweep Spacing"=0, "Range"=0, "SMU1 - Sampling"={"Source"=10.0, "Compliance"=1e-05, "Mode"=0, "Function"=FALSE}, "SMU2 - Sampling"={"Source"=10.0, "Compliance"=1e-05, "Mode"=0, "Function"=FALSE}, "SMU3 - Sampling"={"Source"=10.0, "Compliance"=1e-05, "Mode"=0, "Function"=FALSE}, "SMU4 - Sampling"={"Source"=10.0, "Compliance"=1e-05, "Mode"=0, "Function"=FALSE}, "Sampling Time Parameters"={"Initial Interval (s)"=0.1, "Number of Samples"=60, "Total Sampling Time (s)"=10.0, "Hold Time (s)"=0.0, "Sampling Mode"=0, "Sampling Time"=0}, "Stop Condition"={"Enable Delay (s)"=0.0, "Name"="", "Threshold"=0.0, "num. of events"=1, "Event"=0, "Stop Condition Enable"=FALSE}} ("HP4155C Configuration"), "SMU1 - Sampling"=w409, "SMU2 - Sampling"=w408, "SMU3 - Sampling"=w407, "SMU4 - Sampling"=w406, "Sampling Time Parameters"=w417, "Stop Condition"=w416) -> (w410:T17)
        n188 = Unbundle By Name(w411) -> ("Parameter Analyzer"=w414:refnum<queue>)
        n189 = call "Enqueue Message (Single).vi"("error in (no error)"=w413, "Message Data"=w410, "Message"="Configure Sampling", "Message Queue"=w414) -> ("error out"=w412:errorcluster)  [unwired: 7 out]
      }
      frame "Parameter Analyzer - Save Measurement" {
        n190 = Unbundle By Name(w422) -> ("Parameter Analyzer"=w424:refnum<queue>)
        n191 = call "Enqueue Message (Single).vi"("error in (no error)"=w421, "Message"="Save Electrical Measurement", "Message Queue"=w424) -> ("error out"=w423:errorcluster)  [unwired: 1 in, 7 out]
      }
      frame "----- Switching Matrix Events ----- " {
        # "Switching Matrix Events"
      }
      frame "Switching Matrix - Update Visa Session" {
        w427 = T25 {"Switching Matrix VISA Session"="GPIB0::18::INSTR", "Connections"=[{"Connections"=[FALSE, FALSE, FALSE, FALSE, FALSE, FALSE, FALSE, FALSE, FALSE, FALSE, FALSE, FALSE], "Connection Type"=enum."Disconnected"}, {"Connections"=[FALSE, FALSE, FALSE, FALSE, FALSE, FALSE, FALSE, FALSE, FALSE, FALSE, FALSE, FALSE], "Connection Type"=enum."Disconnected"}, {"Connections"=[FALSE, FALSE, FALSE, FALSE, FALSE, FALSE, FALSE, FALSE, FALSE, FALSE, FALSE, FALSE], "Connection Type"=enum."Disconnected"}, {"Connections"=[FALSE, FALSE, FALSE, FALSE, FALSE, FALSE, FALSE, FALSE, FALSE, FALSE, FALSE, FALSE], "Connection Type"=enum."Disconnected"}, {"Connections"=[FALSE, FALSE, FALSE, FALSE, FALSE, FALSE, FALSE, FALSE, FALSE, FALSE, FALSE, FALSE], "Connection Type"=enum."Disconnected"}, {"Connections"=[FALSE, FALSE, FALSE, FALSE, FALSE, FALSE, FALSE, FALSE, FALSE, FALSE, FALSE, FALSE], "Connection Type"=enum."Disconnected"}, {"Connections"=[FALSE, FALSE, FALSE, FALSE, FALSE, FALSE, FALSE, FALSE, FALSE, FALSE, FALSE, FALSE], "Connection Type"=enum."Disconnected"}, {"Connections"=[FALSE, FALSE, FALSE, FALSE, FALSE, FALSE, FALSE, FALSE, FALSE, FALSE, FALSE, FALSE], "Connection Type"=enum."Disconnected"}]} ("Keythley 707A Switching Matrix Configuration")
        n192 = Unbundle By Name(w427) -> ("Switching Matrix VISA Session"=w428:refnum<visa-resource-name>)
        n193 = Variant To Data(error in=w434, type=w428, Variant=w431) -> (data=w430:refnum<visa-resource-name>, error out=w432:errorcluster)
        n194 = Bundle By Name(cluster=w427, "Switching Matrix VISA Session"=w430) -> (w429:T25)
        n195 = Unbundle By Name(w435) -> ("Switching Matrix"=w436:refnum<queue>)
        n196 = call "Enqueue Message (Single).vi"("error in (no error)"=w432, "Message Data"=w429, "Message"="Update Visa Session", "Message Queue"=w436) -> ("error out"=w437:errorcluster)  [unwired: 7 out]
      }
      frame "Switching Matrix - Set Connections" {
        w438 = T25 {"Switching Matrix VISA Session"="GPIB0::18::INSTR", "Connections"=[{"Connections"=[FALSE, FALSE, FALSE, FALSE, FALSE, FALSE, FALSE, FALSE, FALSE, FALSE, FALSE, FALSE], "Connection Type"=enum."Disconnected"}, {"Connections"=[FALSE, FALSE, FALSE, FALSE, FALSE, FALSE, FALSE, FALSE, FALSE, FALSE, FALSE, FALSE], "Connection Type"=enum."Disconnected"}, {"Connections"=[FALSE, FALSE, FALSE, FALSE, FALSE, FALSE, FALSE, FALSE, FALSE, FALSE, FALSE, FALSE], "Connection Type"=enum."Disconnected"}, {"Connections"=[FALSE, FALSE, FALSE, FALSE, FALSE, FALSE, FALSE, FALSE, FALSE, FALSE, FALSE, FALSE], "Connection Type"=enum."Disconnected"}, {"Connections"=[FALSE, FALSE, FALSE, FALSE, FALSE, FALSE, FALSE, FALSE, FALSE, FALSE, FALSE, FALSE], "Connection Type"=enum."Disconnected"}, {"Connections"=[FALSE, FALSE, FALSE, FALSE, FALSE, FALSE, FALSE, FALSE, FALSE, FALSE, FALSE, FALSE], "Connection Type"=enum."Disconnected"}, {"Connections"=[FALSE, FALSE, FALSE, FALSE, FALSE, FALSE, FALSE, FALSE, FALSE, FALSE, FALSE, FALSE], "Connection Type"=enum."Disconnected"}, {"Connections"=[FALSE, FALSE, FALSE, FALSE, FALSE, FALSE, FALSE, FALSE, FALSE, FALSE, FALSE, FALSE], "Connection Type"=enum."Disconnected"}]} ("Keythley 707A Switching Matrix Configuration")
        n197 = Unbundle By Name(w438) -> ("Connections"=w439:T67)
        n198 = Variant To Data(error in=w445, type=w439, Variant=w442) -> (data=w441:T67, error out=w443:errorcluster)
        n199 = Bundle By Name(cluster=w438, "Connections"=w441) -> (w440:T25)
        n200 = Unbundle By Name(w446) -> ("Switching Matrix"=w447:refnum<queue>)
        n201 = call "Enqueue Message (Single).vi"("error in (no error)"=w443, "Message Data"=w440, "Message"="Set Connections", "Message Queue"=w447) -> ("error out"=w448:errorcluster)  [unwired: 7 out]
      }
      frame "Switching Matrix - Disconnect All" {
        n202 = Unbundle By Name(w451) -> ("Switching Matrix"=w452:refnum<queue>)
        n203 = call "Enqueue Message (Single).vi"("error in (no error)"=w449, "Message"="Disconnect All", "Message Queue"=w452) -> ("error out"=w453:errorcluster)  [unwired: 1 in, 7 out]
      }
      frame "Switching Matrix - Ground All" {
        n204 = Unbundle By Name(w456) -> ("Switching Matrix"=w457:refnum<queue>)
        n205 = call "Enqueue Message (Single).vi"("error in (no error)"=w454, "Message"="Ground All", "Message Queue"=w457) -> ("error out"=w458:errorcluster)  [unwired: 1 in, 7 out]
      }
      frame "----- XYZ Stage Events -----" {
        # "NEW DEVICE EVENTS"
      }
      frame "XYZ Stage - Update Visa Session" {
        w460 = T39 {"Connection Settings"={"Tango VISA"="", "Baudrate"=57600, "Show Protocol?"=FALSE}, "Manual Control"={"North"=FALSE, "South"=FALSE, "West"=FALSE, "East"=FALSE, "Up"=FALSE, "Down"=FALSE, "Stop"=FALSE, "XY Step"=0.0, "Z step"=0.0}, "Coordinate Control"={"Motion Mode"=enum."Absolute", "Destination [mm]"=[]}} ("Configuration")
        n206 = Unbundle By Name(w460) -> ("Connection Settings.Tango VISA"=w468:refnum<visa-resource-name>)
        n207 = Variant To Data(error in=w470, type=w468, Variant=w469) -> (data=w461:refnum<visa-resource-name>, error out=w466:errorcluster)
        n208 = Bundle By Name(cluster=w460, "Connection Settings.Tango VISA"=w461) -> (w462:T39)
        n209 = Unbundle By Name(w464) -> ("XYZ Stage"=w463:refnum<queue>)
        n210 = call "Enqueue Message (Single).vi"("error in (no error)"=w466, "Message Data"=w462, "Message"="Manual Control", "Message Queue"=w463) -> ("error out"=w465:errorcluster)  [unwired: 7 out]
      }
      frame "XYZ Stage - Manual Control" {
        w472 = T39 {"Connection Settings"={"Tango VISA"="", "Baudrate"=57600, "Show Protocol?"=FALSE}, "Manual Control"={"North"=FALSE, "South"=FALSE, "West"=FALSE, "East"=FALSE, "Up"=FALSE, "Down"=FALSE, "Stop"=FALSE, "XY Step"=0.0, "Z step"=0.0}, "Coordinate Control"={"Motion Mode"=enum."Absolute", "Destination [mm]"=[]}} ("Configuration")
        n211 = Unbundle By Name(w472) -> ("Manual Control"=w471:T41)
        n212 = Variant To Data(error in=w481, type=w471, Variant=w480) -> (data=w473:T41, error out=w478:errorcluster)
        n213 = Bundle By Name(cluster=w472, "Manual Control"=w473) -> (w474:T39)
        n214 = Unbundle By Name(w476) -> ("XYZ Stage"=w475:refnum<queue>)
        n215 = call "Enqueue Message (Single).vi"("error in (no error)"=w478, "Message Data"=w474, "Message"="Manual Control", "Message Queue"=w475) -> ("error out"=w477:errorcluster)  [unwired: 7 out]
      }
      frame "----- AutoFocus Events -----" {
        # "NEW DEVICE EVENTS"
      }
      frame "AutoFocus - Set Match Criteria" {
        w483 = T43 {"Matching Criteria"={"Minimum Score"=700.0, "Color Score Weight"=57600.0, "Minimum Contrast"=50, "Match Mode"=0, "Match Feature Mode"=0, "Subpixel Accuracy"=TRUE, "Color Sensitivity"=1, "Search Strategy"=1}, "Z Scan Parameters"={"Z Range"=1380.0, "Resolution"=5000.0, "Initial Direction"=enum."Up", "Focus Threshold"=700.0, "Ascent Constant"=0.1}, "Displacement"=0.0, "Transformation Matrix"=[]} ("Configuration")
        n216 = Unbundle By Name(w483) -> ("Matching Criteria"=w491:T68)
        n217 = Variant To Data(error in=w493, type=w491, Variant=w492) -> (data=w484:T68, error out=w489:errorcluster)
        n218 = Bundle By Name(cluster=w483, "Matching Criteria"=w484) -> (w485:T43)
        n219 = Unbundle By Name(w487) -> ("AutoFocus"=w486:refnum<queue>)
        n220 = call "Enqueue Message (Single).vi"("error in (no error)"=w489, "Message Data"=w485, "Message"="Set Match Criteria", "Message Queue"=w486) -> ("error out"=w488:errorcluster)  [unwired: 7 out]
      }
      frame "AutoFocus - Link Stage & Camera" {
        w494 = T43 {"Matching Criteria"={"Minimum Score"=700.0, "Color Score Weight"=57600.0, "Minimum Contrast"=50, "Match Mode"=0, "Match Feature Mode"=0, "Subpixel Accuracy"=TRUE, "Color Sensitivity"=1, "Search Strategy"=1}, "Z Scan Parameters"={"Z Range"=1380.0, "Resolution"=5000.0, "Initial Direction"=enum."Up", "Focus Threshold"=700.0, "Ascent Constant"=0.1}, "Displacement"=0.0, "Transformation Matrix"=[]} ("Configuration")
        n221 = Unbundle By Name(w494) -> ("Displacement"=w502:dbl)
        n222 = Variant To Data(error in=w504, type=w502, Variant=w503) -> (data=w495:dbl, error out=w500:errorcluster)
        n223 = Bundle By Name(cluster=w494, "Displacement"=w495) -> (w496:T43)
        n224 = Unbundle By Name(w498) -> ("AutoFocus"=w497:refnum<queue>)
        n225 = call "Enqueue Message (Single).vi"("error in (no error)"=w500, "Message Data"=w496, "Message"="Link Stage & Camera", "Message Queue"=w497) -> ("error out"=w499:errorcluster)  [unwired: 7 out]
      }
      frame "AutoFocus - Focus" {
        w505 = T43 {"Matching Criteria"={"Minimum Score"=700.0, "Color Score Weight"=57600.0, "Minimum Contrast"=50, "Match Mode"=0, "Match Feature Mode"=0, "Subpixel Accuracy"=TRUE, "Color Sensitivity"=1, "Search Strategy"=1}, "Z Scan Parameters"={"Z Range"=1380.0, "Resolution"=5000.0, "Initial Direction"=enum."Up", "Focus Threshold"=700.0, "Ascent Constant"=0.1}, "Displacement"=0.0, "Transformation Matrix"=[]} ("Configuration")
        n226 = Unbundle By Name(w505) -> ("Z Scan Parameters"=w513:T44)
        n227 = Variant To Data(error in=w515, type=w513, Variant=w514) -> (data=w506:T44, error out=w511:errorcluster)
        n228 = Bundle By Name(cluster=w505, "Z Scan Parameters"=w506) -> (w507:T43)
        n229 = Unbundle By Name(w509) -> ("AutoFocus"=w508:refnum<queue>)
        n230 = call "Enqueue Message (Single).vi"("error in (no error)"=w511, "Message Data"=w507, "Message"="Focus", "Message Queue"=w508) -> ("error out"=w510:errorcluster)  [unwired: 7 out]
      }
      frame "AutoFocus - Set Target" {
        n231 = Unbundle By Name(w518) -> ("AutoFocus"=w517:refnum<queue>)
        n232 = call "Enqueue Message (Single).vi"("error in (no error)"=w516, "Message"="Set Target", "Message Queue"=w517) -> ("error out"=w519:errorcluster)  [unwired: 1 in, 7 out]
      }
      frame "AutoFocus - Find Target" {
        n233 = Unbundle By Name(w523) -> ("AutoFocus"=w522:refnum<queue>)
        n234 = call "Enqueue Message (Single).vi"("error in (no error)"=w521, "Message"="Find Target", "Message Queue"=w522) -> ("error out"=w524:errorcluster)  [unwired: 1 in, 7 out]
      }
      frame "AutoFocus - Align" {
        n235 = Unbundle By Name(w528) -> ("AutoFocus"=w527:refnum<queue>)
        n236 = call "Enqueue Message (Single).vi"("error in (no error)"=w526, "Message"="Align", "Message Queue"=w527) -> ("error out"=w529:errorcluster)  [unwired: 1 in, 7 out]
      }
      frame "AutoFocus - Grab Image" {
        n237 = Unbundle By Name(w533) -> ("AutoFocus"=w532:refnum<queue>)
        n238 = call "Enqueue Message (Single).vi"("error in (no error)"=w531, "Message"="Grab Image", "Message Queue"=w532) -> ("error out"=w534:errorcluster)  [unwired: 1 in, 7 out]
      }
      frame "AutoFocus - Set ROI" {
        n239 = Unbundle By Name(w538) -> ("AutoFocus"=w537:refnum<queue>)
        n240 = call "Enqueue Message (Single).vi"("error in (no error)"=w536, "Message"="Set ROI", "Message Queue"=w537) -> ("error out"=w539:errorcluster)  [unwired: 1 in, 7 out]
      }
      frame "AutoFocus - Get ROI" {
        n241 = Unbundle By Name(w543) -> ("AutoFocus"=w542:refnum<queue>)
        n242 = call "Enqueue Message (Single).vi"("error in (no error)"=w541, "Message"="Get ROI", "Message Queue"=w542) -> ("error out"=w544:errorcluster)  [unwired: 1 in, 7 out]
      }
      frame "AutoFocus - Start Tracking" {
        n243 = Unbundle By Name(w548) -> ("AutoFocus"=w547:refnum<queue>)
        n244 = call "Enqueue Message (Single).vi"("error in (no error)"=w546, "Message"="Start Tracking", "Message Queue"=w547) -> ("error out"=w549:errorcluster)  [unwired: 1 in, 7 out]
      }
      frame "AutoFocus - Stop Tracking" {
        n245 = Unbundle By Name(w553) -> ("AutoFocus"=w552:refnum<queue>)
        n246 = call "Enqueue Message (Single).vi"("error in (no error)"=w551, "Message"="Stop Tracking", "Message Queue"=w552) -> ("error out"=w554:errorcluster)  [unwired: 1 in, 7 out]
      }
      frame "----- Instrument Sequence Events -----" {
        # "NEW DEVICE EVENTS"
      }
      frame "Instrument Sequence - Add Step" {
        n247 = Unbundle By Name(w561) -> ("Instrument Sequence"=w560:refnum<queue>)
        n248 = call "Enqueue Message (Single).vi"("error in (no error)"=w559, "Message"="Add Step", "Message Queue"=w560) -> ("error out"=w558:errorcluster)  [unwired: 1 in, 7 out]
      }
      frame "Instrument Sequence - Remove Step" {
        n249 = Unbundle By Name(w566) -> ("Instrument Sequence"=w565:refnum<queue>)
        n250 = call "Enqueue Message (Single).vi"("error in (no error)"=w564, "Message"="Remove Step", "Message Queue"=w565) -> ("error out"=w563:errorcluster)  [unwired: 1 in, 7 out]
      }
      frame "Instrument Sequence - Clear Sequence" {
        n251 = Unbundle By Name(w571) -> ("Instrument Sequence"=w570:refnum<queue>)
        n252 = call "Enqueue Message (Single).vi"("error in (no error)"=w569, "Message"="Clear Sequence", "Message Queue"=w570) -> ("error out"=w568:errorcluster)  [unwired: 1 in, 7 out]
      }
      frame "Instrument Sequence - Save Sequence" {
        n253 = Unbundle By Name(w576) -> ("Instrument Sequence"=w575:refnum<queue>)
        n254 = call "Enqueue Message (Single).vi"("error in (no error)"=w574, "Message"="Save Sequence", "Message Queue"=w575) -> ("error out"=w573:errorcluster)  [unwired: 1 in, 7 out]
      }
      frame "Instrument Sequence - Load Sequence" {
        n255 = Unbundle By Name(w581) -> ("Instrument Sequence"=w580:refnum<queue>)
        n256 = call "Enqueue Message (Single).vi"("error in (no error)"=w579, "Message"="Load Sequence", "Message Queue"=w580) -> ("error out"=w578:errorcluster)  [unwired: 1 in, 7 out]
      }
      frame "Instrument Sequence - Start Sequence" {
        n257 = Unbundle By Name(w586) -> ("Instrument Sequence"=w585:refnum<queue>)
        n258 = call "Enqueue Message (Single).vi"("error in (no error)"=w582, "Message"="Start Sequence", "Message Queue"=w585) -> ("error out"=w584:errorcluster)  [unwired: 1 in, 7 out]
      }
      frame "Instrument Sequence - Stop Sequence" {
        n259 = Unbundle By Name(w591) -> ("Instrument Sequence"=w590:refnum<queue>)
        n260 = call "Enqueue Message (Single).vi"("error in (no error)"=w587, "Message"="Measure Sequence", "Message Queue"=w590) -> ("error out"=w589:errorcluster)  [unwired: 1 in, 7 out]
      }
      frame "Instrument Sequence - Pause Sequence" {
        n261 = Unbundle By Name(w596) -> ("Instrument Sequence"=w595:refnum<queue>)
        n262 = call "Enqueue Message (Single).vi"("error in (no error)"=w592, "Message"="Pause Sequence", "Message Queue"=w595) -> ("error out"=w594:errorcluster)  [unwired: 1 in, 7 out]
      }
      frame "----- StrainElectrical Measurement Events -----" {
        # "NEW DEVICE EVENTS"
      }
      frame "Strain Measurement - Update Strain Sequence" {
        w598 = T58 {"Stress Sequence "={"Max Motor Position"=1380.0, "# Intermediate Points"=5000, "Initial Direction"=enum."Tension"}, "Track?"=FALSE} ("Strain Measurement")
        n263 = Unbundle By Name(w598) -> ("Stress Sequence"=w599:T69)
        n264 = Variant To Data(error in=w608, type=w599, Variant=w607) -> (data=w601:T69, error out=w606:errorcluster)
        n265 = Bundle By Name(cluster=w598, "Stress Sequence"=w601) -> (w600:T58)
        n266 = Unbundle By Name(w602) -> ("Strain Measurement"=w603:refnum<queue>)
        n267 = call "Enqueue Message (Single).vi"("error in (no error)"=w606, "Message Data"=w600, "Message"="Define Strain Sequence", "Message Queue"=w603) -> ("error out"=w605:errorcluster)  [unwired: 7 out]
      }
      frame "Strain Measurement - Start" {
        n268 = Unbundle By Name(w609) -> ("Strain Measurement"=w610:refnum<queue>)
        n269 = call "Enqueue Message (Single).vi"("error in (no error)"=w613, "Message"="Start Strain Measurement", "Message Queue"=w610) -> ("error out"=w612:errorcluster)  [unwired: 1 in, 7 out]
      }
      frame "Strain Measurement - Pause" {
        n270 = Unbundle By Name(w614) -> ("Strain Measurement"=w615:refnum<queue>)
        n271 = call "Enqueue Message (Single).vi"("error in (no error)"=w618, "Message"="Pause", "Message Queue"=w615) -> ("error out"=w617:errorcluster)  [unwired: 1 in, 7 out]
      }
      frame "Strain Measurement - Stop" {
        n272 = Unbundle By Name(w619) -> ("Strain Measurement"=w620:refnum<queue>)
        n273 = call "Enqueue Message (Single).vi"("error in (no error)"=w623, "Message"="Stop", "Message Queue"=w620) -> ("error out"=w622:errorcluster)  [unwired: 1 in, 7 out]
      }
      frame "Strain Measurement - New Sequence" {
        n274 = Unbundle By Name(w628) -> ("Strain Measurement"=w627:refnum<queue>)
        n275 = call "Enqueue Message (Single).vi"("error in (no error)"=w626, "Message"="Clear Instrument Sequence", "Message Queue"=w627) -> ("error out"=w625:errorcluster)  [unwired: 1 in, 7 out]
      }
      frame "Strain Measurement - Add Step" {
        n276 = Unbundle By Name(w633) -> ("Strain Measurement"=w632:refnum<queue>)
        n277 = call "Enqueue Message (Single).vi"("error in (no error)"=w631, "Message"="Add Instrument Sequence Step", "Message Queue"=w632) -> ("error out"=w630:errorcluster)  [unwired: 1 in, 7 out]
      }
      frame "Strain Measurement - Delete Step" {
        n278 = Unbundle By Name(w638) -> ("Strain Measurement"=w637:refnum<queue>)
        n279 = call "Enqueue Message (Single).vi"("error in (no error)"=w636, "Message"="Delete Instrument Sequence Step", "Message Queue"=w637) -> ("error out"=w635:errorcluster)  [unwired: 1 in, 7 out]
      }
      frame "Strain Measurement - Save Sequence" {
        n280 = Unbundle By Name(w643) -> ("Strain Measurement"=w642:refnum<queue>)
        n281 = call "Enqueue Message (Single).vi"("error in (no error)"=w641, "Message"="Save Instrument Sequence", "Message Queue"=w642) -> ("error out"=w640:errorcluster)  [unwired: 1 in, 7 out]
      }
      frame "Strain Measurement - Load Sequence" {
        n282 = Unbundle By Name(w648) -> ("Strain Measurement"=w647:refnum<queue>)
        n283 = call "Enqueue Message (Single).vi"("error in (no error)"=w646, "Message"="Load Instrument Sequence", "Message Queue"=w647) -> ("error out"=w645:errorcluster)  [unwired: 1 in, 7 out]
      }
      frame "----- PlotData Events -----" {
        # "NEW DEVICE EVENTS"
      }
      frame "PlotData - Update Plots" {
        n284 = Variant To Data(error in=w662, type=T62 {"PlotData - Instrument Sequence"=0, "PlotData - Strain Sequence"=0} ("output cluster"), Variant=w661) -> (data=w653:T62, error out=w658:errorcluster)
        n285 = Unbundle By Name(w653) -> ("PlotData - Strain Sequence"=w652:i32, "PlotData - Instrument Sequence"=w651:i32)
        n286 = Bundle By Name(cluster=T51 {"Sliders"={"Strain Sequence"=0, "Instrument Sequence"=0}, "Measurement"={"Which Instrument?"=enum."No Plot", "Electrical Measurement"={"Sequence"=[], "V1"=[], "V2"=[], "V3"=[], "V4"=[], "I1"=[], "I2"=[], "I3"=[], "I4"=[]}, "Measurement Mode"=enum."Sweeping Mode", "Optical Spectrum"={"Intensity"=[], "Wavelength"=[], "Energy"=[], "Raman Shift"=[], "Detector Temperature"=0.0}}, "Instrument Steps"=[], "Strain Points"=[]} ("PlotData Configuration"), "Sliders.Strain Sequence"=w652, "Sliders.Instrument Sequence"=w651) -> (w655:T51)
        n287 = Unbundle By Name(w656) -> ("Plot Data"=w659:refnum<queue>)
        n288 = call "Enqueue Message (Single).vi"("error in (no error)"=w658, "Message Data"=w655, "Message"="Plot Data", "Message Queue"=w659) -> ("error out"=w657:errorcluster)  [unwired: 7 out]
      }
      frame "----- Save Data Events -----" {
        # "Save Data Events"
      }
    }
    n289 = call "Message Handling Loop.vi"("error in (no error)"=w38, "Message Queue"=w36) -> ("dup error in"=w37:errorcluster)  [unwired: 9 out]
  }
  n290 = while "Event Handling Loop" {
    tunnel: w24 -> [w670]
    tunnel: [w669] -> w23
    tunnel: w22 -> [w667]
    tunnel: [w665] -> w21
    stop <- w664 stop-if-true
    n291 = event shown="[6] \"Laser\": Value Change" {
      selector: w670 -> [_ _ _ _ _ _ _]
      dyn-events: [_ _ _ _ _ _ _] -> w665
      timeout: _ -> [_ _ _ _ _ _ _]
      tunnel: [w672 _ w680 _ w690 w695 w711] -> w668
      tunnel: w667 -> [w675 w677 w682 w687 w693 w700 w715]
      tunnel: [w671 w677 w681 w687 w692 w697 w712] -> w666
      tunnel: [_ _ _ TRUE ("Priority Message? (F)") _ _ _] -> w664
      event Panel Close? {
        # "Send the \"Confirm Quit\" message if the user closes the panel of the VI. Discard the event so the \"Confirm Quit\" message has a chance to run."
        n292 = event-data() -> ()  [unwired: 2 out]
        n293 = call "Enqueue Message (Single).vi"("Priority Message? (F)"=TRUE, "Message"="Initiate Exit", "Message Queue"=w675) -> ("error out"=w672:errorcluster, "dup Message Queue"=w671:refnum<queue>)  [unwired: 2 in, 5 out]
        n294 = event-data("Discard?"=TRUE) -> ()  [unwired: 1 in, 1 out]
      }
      event Application Instance Close {
        # "#CodeRecommended - When a project closes, all VIs within that project are aborted and leave memory. However, any code placed in this event frame is guaranteed to run to completion, so add any cleanup code that absolutely must happen here."
        n295 = event-data() -> ()  [unwired: 2 out]
      }
      event "Exit": Value Change {
        n296 = event-data() -> ()  [unwired: 2 out]
        n297 = call "Enqueue Message (Single).vi"("Priority Message? (F)"=TRUE, "Message"="Initiate Exit", "Message Queue"=w682) -> ("error out"=w680:errorcluster, "dup Message Queue"=w681:refnum<queue>)  [unwired: 2 in, 5 out]
      }
      event User Event {
        n298 = event-data() -> ()  [unwired: 2 out]
        n299 = call "Status String.vi"("Message"="Program Terminated" ("Display <Replace Me>")) -> ("Status String"=w683:string)
        n300 = property on="Status Log" class="Str"() -> ("Value"=w685:string)  [unwired: 2 in, 2 out]
        n301 = Concatenate Strings(w683, w685) -> (w686:string)
        n302 = property on="Status Log" class="Str"("Value"=w686) -> ()  [unwired: 2 in, 2 out]
      }
      event "Switches & Mirrors VISA Session": Value Change {
        n303 = event-data() -> ()  [unwired: 2 out]
        n304 = call "Enqueue Message (Single).vi"("Message Data"="Switches & Mirrors VISA Session", "Message"="Switches & Mirrors - Update Visa Session", "Message Queue"=w693) -> ("error out"=w690:errorcluster, "dup Message Queue"=w692:refnum<queue>)  [unwired: 1 in, 6 out]
      }
      event "Video": Value Change {
        n305 = event-data() -> ()  [unwired: 2 out]
        n306 = call "Enqueue Message (Single).vi"("Message Data"="Video", "Message"="Switches & Mirrors - Update Video", "Message Queue"=w700) -> ("error out"=w696:errorcluster, "dup Message Queue"=w698:refnum<queue>)  [unwired: 1 in, 6 out]
        n307 = case shown="True" "Video" {
          tunnel: w698 -> [w704 w709]
          tunnel: [w703 w708] -> w697
          tunnel: w696 -> [w702 w707]
          tunnel: [w701 w706] -> w695
          frame True {
            n308 = call "Enqueue Message (Single).vi"("error in (no error)"=w702, "Message"="Camera - Start Live", "Message Queue"=w704) -> ("error out"=w701:errorcluster, "dup Message Queue"=w703:refnum<queue>)  [unwired: 1 in, 6 out]
          }
          frame False {
            n309 = call "Enqueue Message (Single).vi"("error in (no error)"=w707, "Message"="Camera - Stop Live", "Message Queue"=w709) -> ("error out"=w706:errorcluster, "dup Message Queue"=w708:refnum<queue>)  [unwired: 1 in, 6 out]
          }
        }
      }
      event "Laser": Value Change {
        n310 = event-data() -> ()  [unwired: 2 out]
        n311 = call "Enqueue Message (Single).vi"("Message Data"="Laser", "Message"="Switches & Mirrors - Update Laser", "Message Queue"=w715) -> ("error out"=w711:errorcluster, "dup Message Queue"=w712:refnum<queue>)  [unwired: 1 in, 6 out]
      }
    }
    n312 = call "Event Handling Loop.vi"("error in (no error)"=w668, "Message Queue"=w666) -> ("dup error in"=w669:errorcluster)  [unwired: 9 out]
  }
  n313 = Send Notification(notification=TRUE, notifier=w3, error in (no error)=w5) -> (error out=w1:errorcluster)  [unwired: 1 out]
  n314 = Unregister For Events(event registration refnum=w21, error in=w23) -> (error out=w9:errorcluster)
  n315 = Merge Errors(w9, w8, w7, w1) -> (w16:errorcluster)
  n316 = call "Close Notifiers.vi"("error in"=w16, "Notifiers"=w4) -> ("error out"=w15:errorcluster)  [unwired: 9 out]
  n317 = call "Destroy User Event - Stop.vi"("error in (no error)"=w15, "User Event - Stop"=w17) -> ("error out"=w20:errorcluster)  [unwired: 9 out]
  n318 = property class="App"(error in=w20) -> (error out=w18:errorcluster, "App.Kind"=w19:T70)  [unwired: 1 in, 1 out]
  n319 = case shown="\"Development System\"" w19 {
    tunnel: w18 -> [w716 w717 _ _ _ _ _]
    frame "invalid app kind", Default {
      n320 = call <vilib>:"Simple Error Handler.vi"("error in (no error)"=w716) -> ()  [unwired: 1 in, 8 out]
    }
    frame "Development System" {
      n321 = call <vilib>:"Simple Error Handler.vi"("error in (no error)"=w717) -> ()  [unwired: 1 in, 8 out]
    }
    frame "Run Time System" {
      n322 = Quit LabVIEW() -> ()  [unwired: 1 out]
    }
    frame "Student Edition" {
    }
    frame "Embedded LabVIEW" {
    }
    frame "Evaluation" {
    }
    frame "Custom" {
    }
  }
